vi "运维调试_五参数.vi"() -> ()   [LabVIEW 2016, in "斯坦道多参数.lvlib"]
uses:
  <vilib>/Utility/miscctls.llb/LVPointTypeDef.ctl
  <vilib>/Utility/config.llb/NI_LVConfig.lvlib
panel:
  in  "获取传感器参数并保存触发":bool
  in  "传感器参数自动获取":bool=TRUE
  in  "标样测试组数":dbl=1.0 caption="标样测试组数:"
  in  "水样测试组数":dbl=1.0 caption="水样测试组数:"
  in  "转刷清洗时间":dbl=30.0 caption="转刷清洗时间:"
  in  "上电初始化时间":dbl=5.0 caption="上电初始化时间:"
  in  "水样稳定时间":dbl=5.0 caption="水样稳定时间:"
  out "串口号":string
  in  "水深写入":bool
  in  "水深读取":bool
  in  "水深校准":dbl caption="水深校准:"
  in  "仪器参数设置":bool
  out "模块版本号":string
  in  "写入":bool
  in  "读取":bool
  in  "B":dbl caption="校准值B:"
  in  "K":dbl caption="校准值K:"
  in  "标样核查":bool
  in  "串口设置":bool
  in  "质控参数设置":bool
  in  "打开串口":bool
  in  "释放串口":bool
  out "多参数横条运行状态":T1(xcontrol)
  in  "数据区":i32(listbox)
  in  "停止测量(单探)":bool
  in  "启动测量(单探)":bool
  in  "控制命令区探头选择":u16(ring)=9 items=["氨氮"=3, "水温"=9, "pH值"=10, "溶解氧"=11, "电导率"=12, "浊度"=13, "叶绿素a"=14, "藻密度"=15, "蓝绿藻"=16, "氧化还原电位"=17, "溶解氧%"=18, "盐度"=19]
  in  "同步时间":bool
  in  "初始化(清洗)":bool
  in  "停止测量(全部)":bool
  in  "启动测量(全部)":bool
  in  "关键参数区读取":bool
  in  "关键参数区":i32(listbox)
  in  "传感器参数读取":bool
  in  "传感器区":i32(listbox)
  in  "返回":bool
  in  "设置":bool
  out "运行状态":string
  in  "停止":bool
  in  "水样测试":bool
  out "集成报警信息":string
  # "min"
  # "组"
  # "组"
  # "s"
  # "s"
  # "控制命令区"
  # "探头校准"
  # "水深校准"
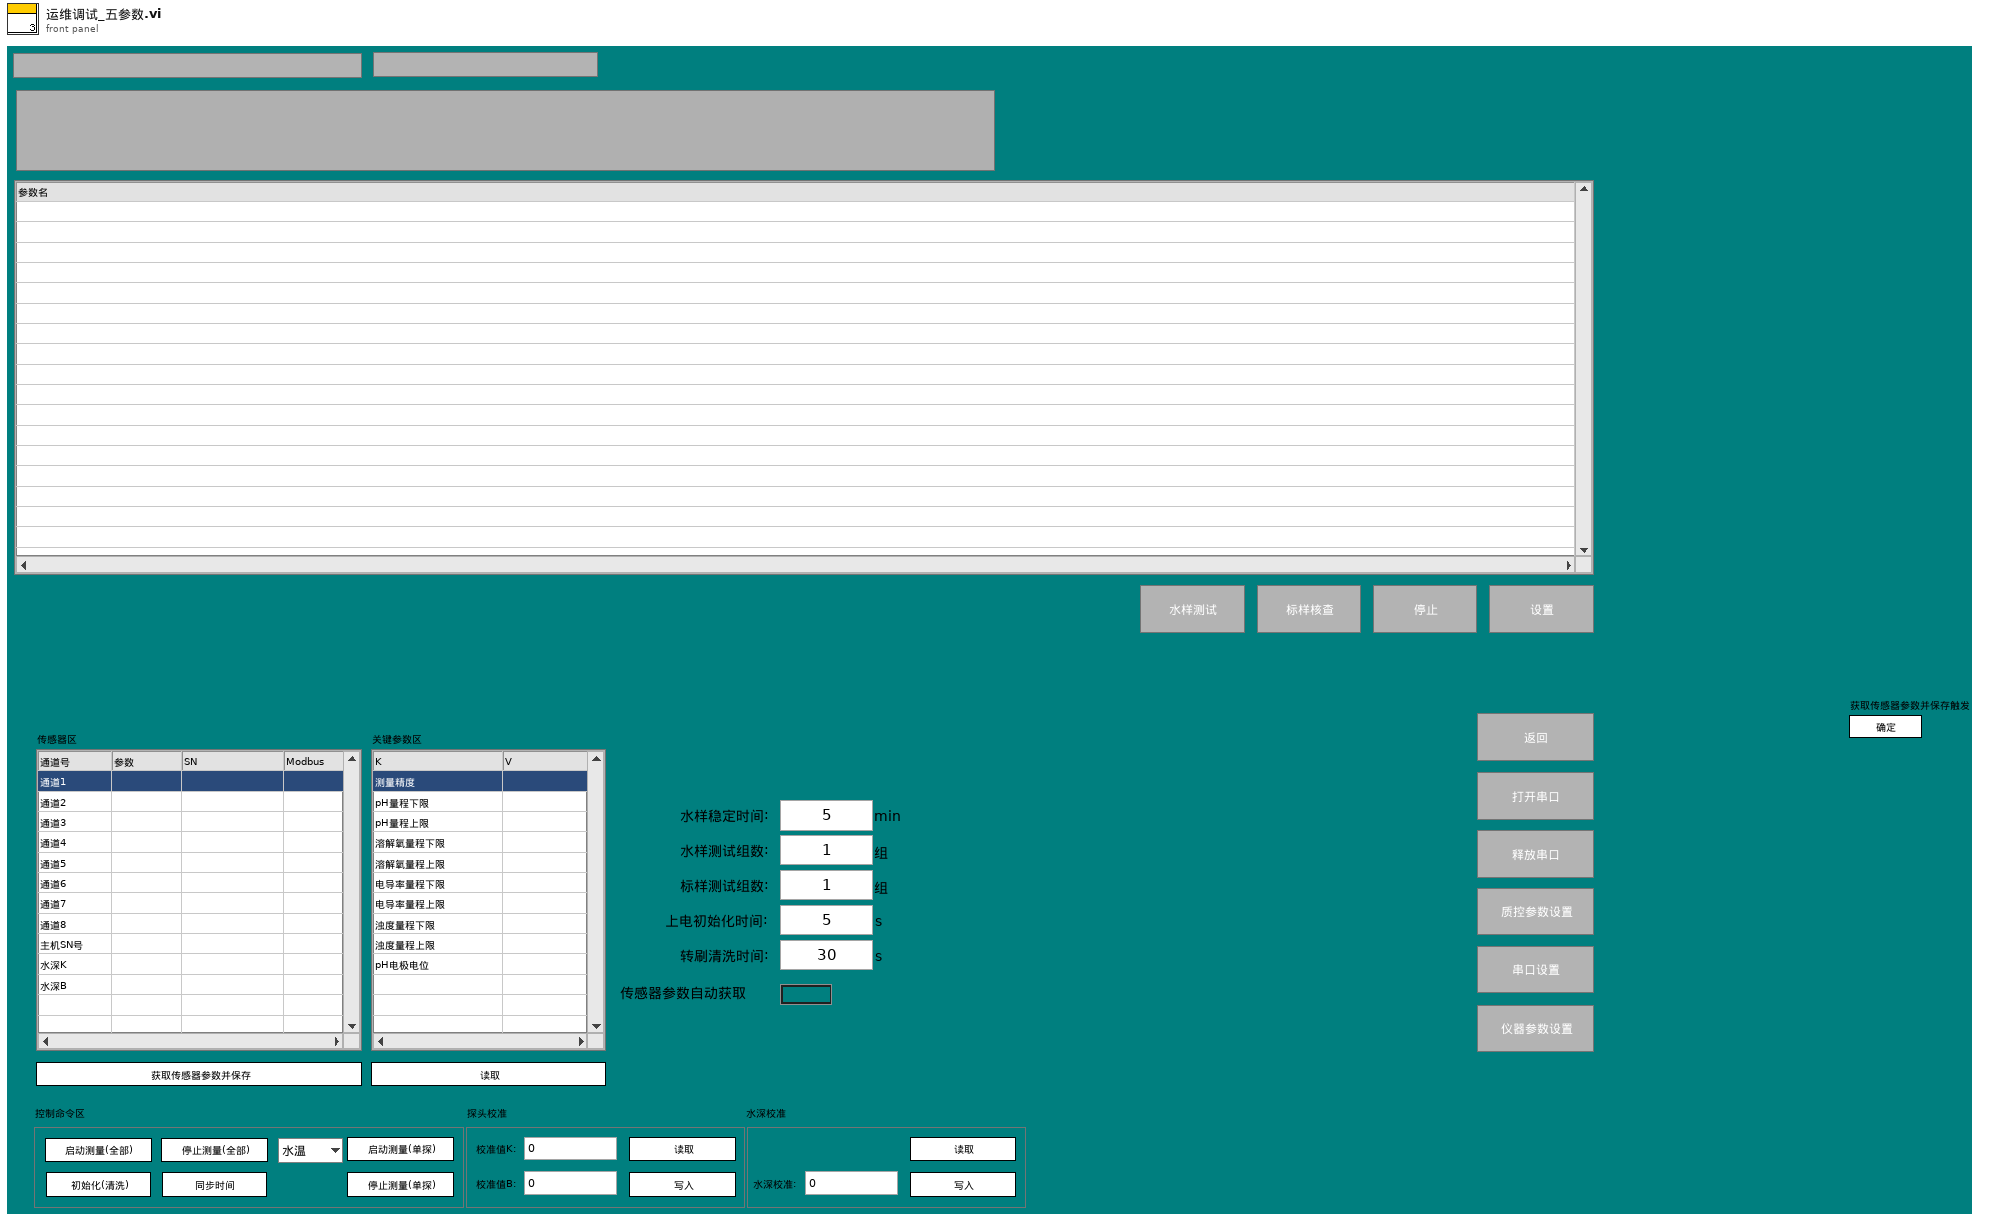
[diagram p1: front panel]
types:
  T1 = cluster{"系统时间":timestamp, "工作状态":u16, "测量模式":u16, "告警代码":enum16{"无告警", "缺试剂告警", "缺水样告警", "缺蒸馏水告警", "缺标液告警", "仪表漏液告警", "标定异常告警", "超量程告警", "加热异常", "低试剂预警", "超上限告警", "超下限告警", "仪表内部其他异常", "滴定异常告警", "电极异常告警", "量程切换告警", "参数设置告警", "PH电极电位异常", "电导率电极异常", "浊度光度异常", "溶解氧电极异常", "溶解氧光强异常", "温度异常告警", "PH异常告警", "溶解氧异常告警", "电导率异常告警", "浊度异常告警", "叶绿素异常告警", "藻密度异常告警", "蓝绿藻异常告警", "ORP异常告警", "氨氮异常告警", "清洁刷异常告警", "SD卡异常告警", "蓝牙异常告警", "Wifi异常告警", "流程异常告警"}, "故障代码":enum16{"无故障", "电机故障", "温度故障", "通讯故障", "滴定故障"}, "日志代码":u16, "软件版本":string}
  T2 = typedef "斯坦道多参数.lvlib/水样测试启动自定义输入参数.ctl" = cluster{"测量模式":enum16{"待机", "水样测试", "标样核查", "零点核查", "跨度核查", "空白测试", "平行样测试", "加标回收", "空白校准", "标样校准", "初始化（清洗）"}, "数据类型":string, "手动启动标记":bool}
  T3 = typedef "LVPointTypeDef.ctl" = cluster{"Horizontal":i16, "Vertical":i16}
  T4 = cluster{"测量量程":dbl, "测量精度":dbl, "测量间隔":dbl, "消解温度":dbl, "消解时长":dbl, "空白校准时间":timestamp, "曲线截距":dbl, "曲线斜率":dbl, "测量检出限":dbl, "测量信号值":dbl, "线性相关系数":dbl, "二次多项式系数":dbl, "标样校准时间":timestamp, "稀释倍数":dbl, "三项式系数":dbl, "空白标定系数":dbl, "量程系数":dbl, "F0/ORPA":dbl, "F1/ORPB":dbl, "F2/ORPK":dbl, "F3":dbl, "F4":dbl, "F5":dbl, "F6":dbl, "F7":dbl, "X0/滴定数":dbl, "量程":dbl}
  T5 = cluster{"因子编码":string, "单位":string, "标样参考值":sgl, "水样数据时间":timestamp, "水样实测值":sgl, "水样数据标识":string, "K":sgl, "B":sgl, "T":sgl, "H":sgl, "水深":sgl, "探头温度":sgl}
  T6 = cluster{"测量量程":dbl, "测量精度":dbl, "测量间隔":dbl, "消解温度":dbl, "消解时长":dbl, "空白校准时间":timestamp, "曲线截距":dbl, "曲线斜率":dbl, "测量检出限":dbl, "测量信号值":dbl, "线性相关系数":dbl, "二次多项式系数":dbl, "标样校准时间":timestamp, "稀释倍数":dbl, "三项式系数":dbl, "空白标定系数":dbl, "量程系数":dbl, "F0/ORPA":dbl, "F1/ORPB":dbl, "F2/ORPK":dbl, "F3":dbl, "F4":dbl, "F5":dbl, "F6":dbl, "F7":dbl, "X0/滴定数":dbl, "量程":dbl}[]
  T7 = cluster{"因子编码":string, "单位":string, "标样参考值":sgl, "水样数据时间":timestamp, "水样实测值":sgl, "水样数据标识":string, "K":sgl, "B":sgl, "T":sgl, "H":sgl, "水深":sgl, "探头温度":sgl}[]
  T8 = cluster{"时间标识":timestamp, "设备":string, "日志信息":string}
  T9 = enum16{"无告警", "缺试剂告警", "缺水样告警", "缺蒸馏水告警", "缺标液告警", "仪表漏液告警", "标定异常告警", "超量程告警", "加热异常", "低试剂预警", "超上限告警", "超下限告警", "仪表内部其他异常", "滴定异常告警", "电极异常告警", "量程切换告警", "参数设置告警", "PH电极电位异常", "电导率电极异常", "浊度光度异常", "溶解氧电极异常", "溶解氧光强异常", "温度异常告警", "PH异常告警", "溶解氧异常告警", "电导率异常告警", "浊度异常告警", "叶绿素异常告警", "藻密度异常告警", "蓝绿藻异常告警", "ORP异常告警", "氨氮异常告警", "清洁刷异常告警", "SD卡异常告警", "蓝牙异常告警", "Wifi异常告警", "流程异常告警"}
  T10 = cluster{"水温":dbl, "pH":dbl, "DO":dbl, "Cond":dbl, "Turb":dbl, "叶绿素":dbl, "藻密度":dbl, "蓝绿藻":dbl, "ORP":dbl, "NH3N":dbl}
  T11 = cluster{"Major":u16, "Minor":u16, "Fix":u16, "Build":u16}
  T12 = typedef "NI_LVConfig.lvlib/Config Data RefNum.ctl" = refnum<k1>
  T13 = enum8{"Enabled", "Disabled", "Disabled and Grayed Out"}
  T14 = typedef "斯坦道多参数.lvlib/标样核查启动自定义输入参数.ctl" = cluster{"测量模式":enum16{"待机", "水样测试", "标样核查", "零点核查", "跨度核查", "空白测试", "平行样测试", "加标回收", "空白校准", "标样校准", "初始化（清洗）"}, "数据标记表":string, "输出参数":cluster{"水温":bool, "pH":bool, "DO":bool, "浊度":bool, "电导率":bool}}
  T15 = cluster{"水温标准液标准浓度":dbl, "酸碱度标准液标准浓度":dbl, "溶解氧标准液标准浓度":dbl, "电导率标准液标准浓度":dbl, "浊度标准液标准浓度":dbl}
  T16 = cluster{"确定":bool, "水温标准液标准浓度":dbl, "酸碱度标准液标准浓度":dbl, "溶解氧标准液标准浓度":dbl, "电导率标准液标准浓度":dbl, "浊度标准液标准浓度":dbl}
  T17 = cluster{"运行模式":enum16{"维护模式", "常规模式", "应急模式", "质控模式"}, "24H周期设置":bool[]}
  T18 = cluster{"水温":bool, "pH":bool, "DO":bool, "浊度":bool, "电导率":bool}
  T19 = enum32{"Bad", "Idle", "Run top level", "Running"}
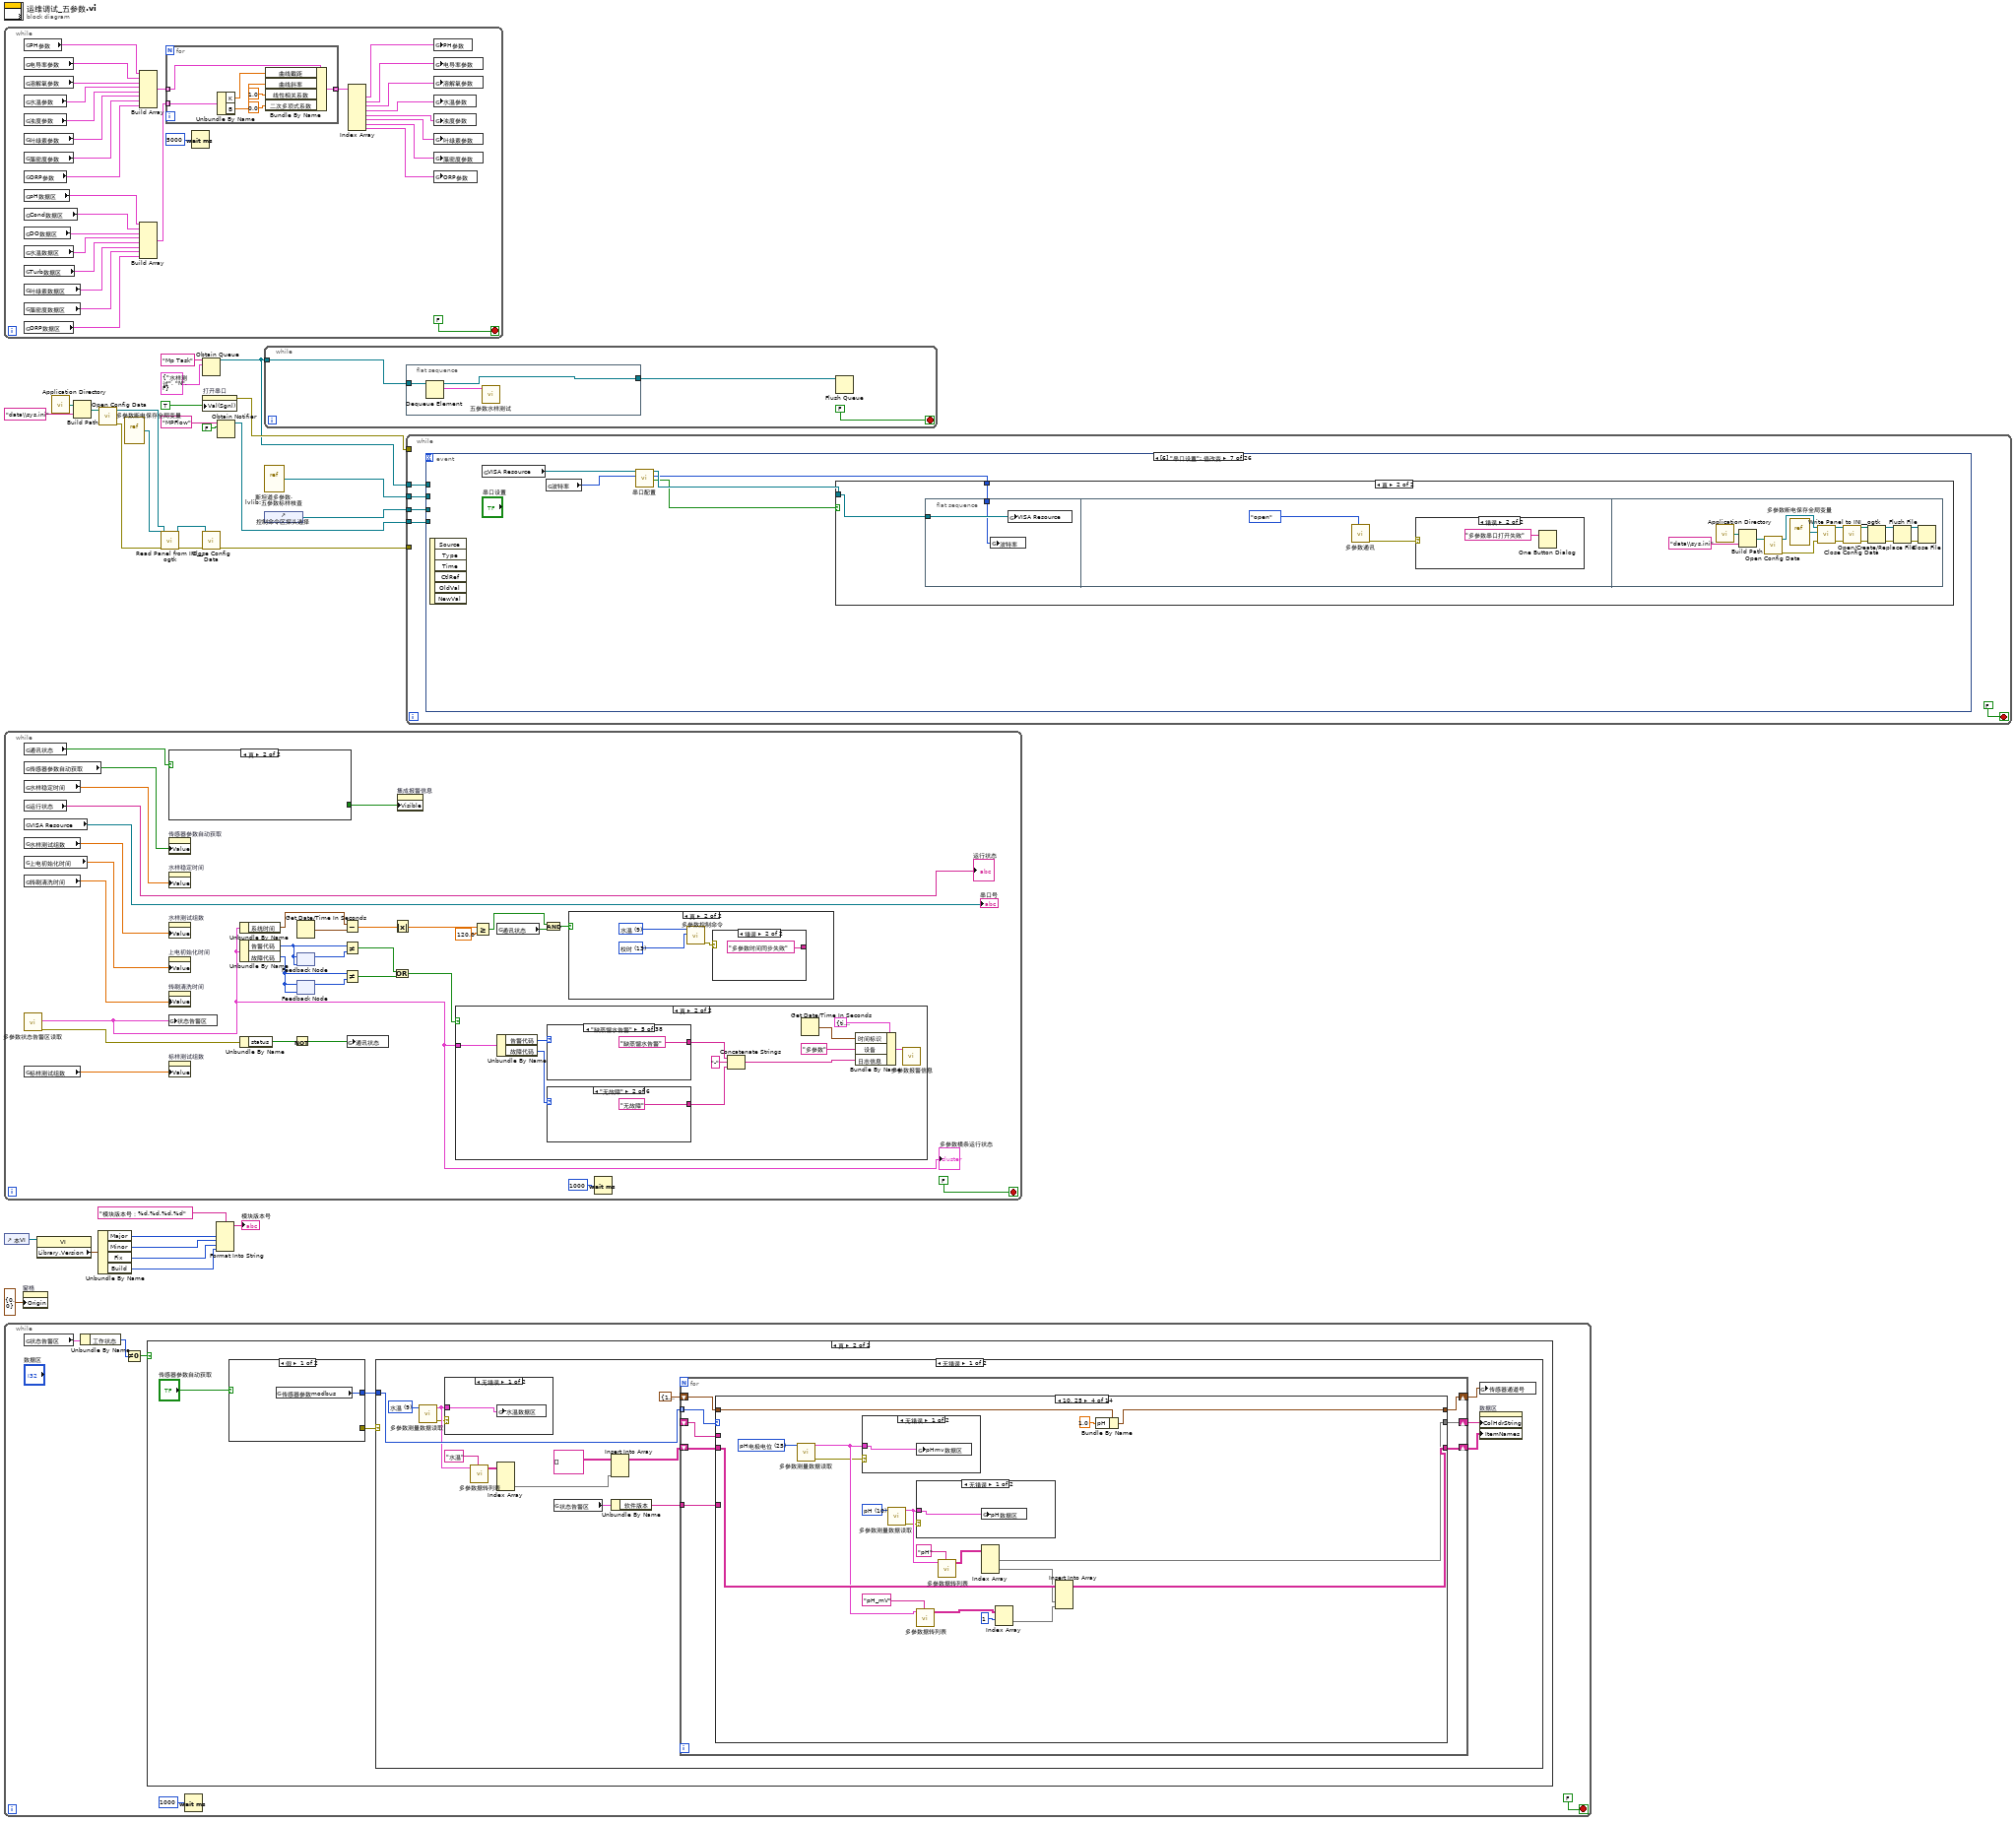
[diagram p0: block diagram]
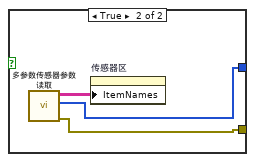
[diagram p3: hidden frame]
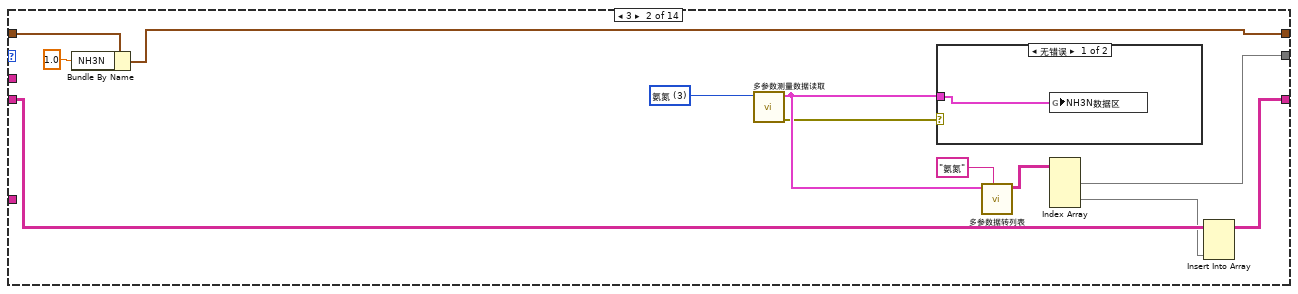
[diagram p6: hidden frame]
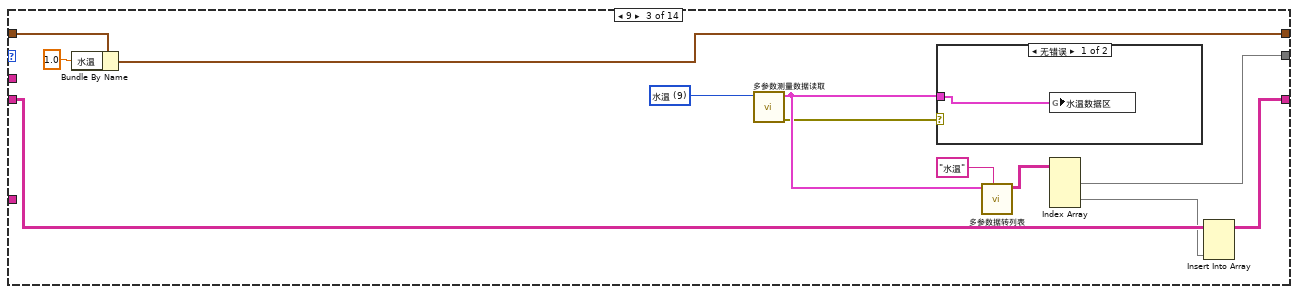
[diagram p8: hidden frame]
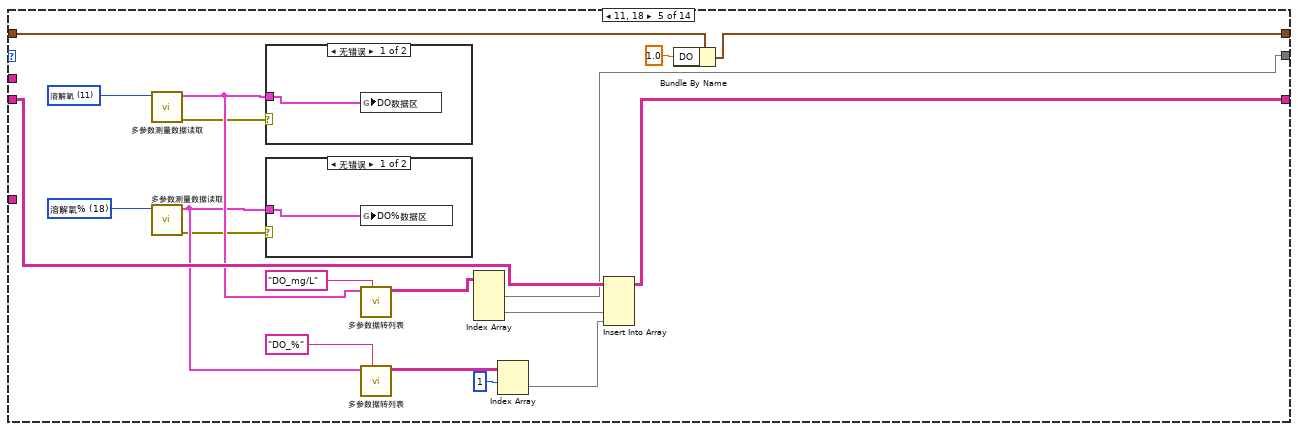
[diagram p12: hidden frame]
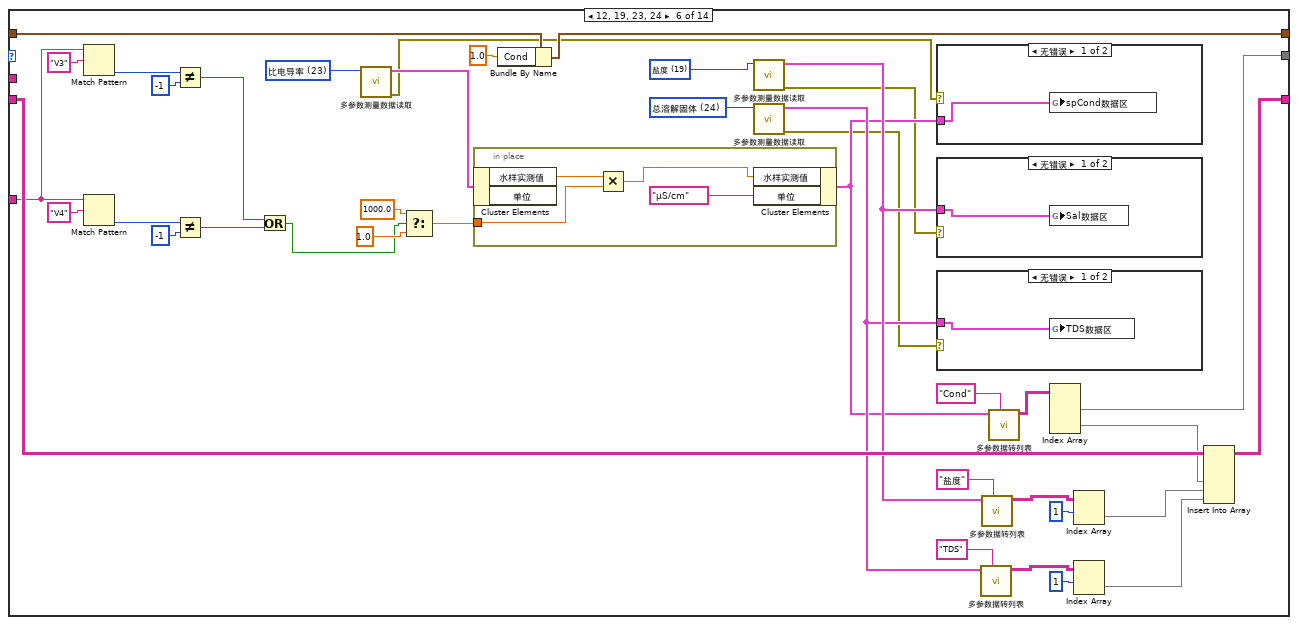
[diagram p15: hidden frame]
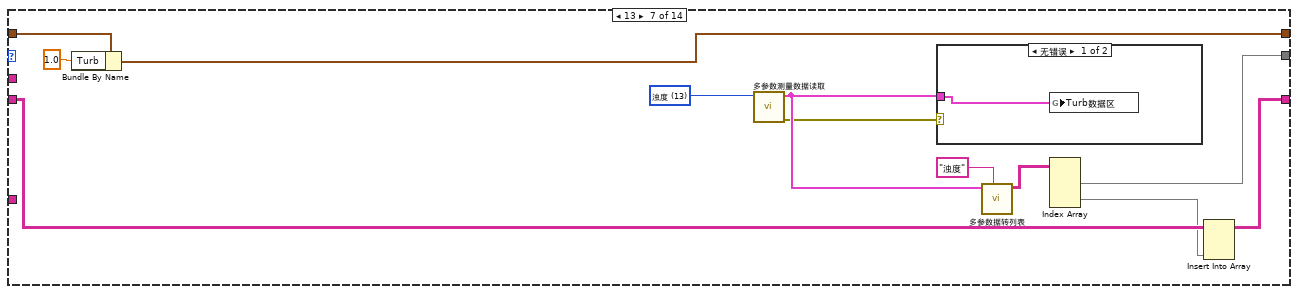
[diagram p19: hidden frame]
diagram:
  n1 = while {
    stop <- FALSE stop-if-true
    n2 = global read "多参数断电保存全局变量.vi" "PH参数"() -> (w47:T4)
    n3 = global read "多参数断电保存全局变量.vi" "电导率参数"() -> (w46:T4)
    n4 = global read "多参数断电保存全局变量.vi" "溶解氧参数"() -> (w45:T4)
    n5 = global read "多参数断电保存全局变量.vi" "水温参数"() -> (w44:T4)
    n6 = global read "多参数断电保存全局变量.vi" "浊度参数"() -> (w43:T4)
    n7 = global read "多参数断电保存全局变量.vi" "叶绿素参数"() -> (w42:T4)
    n8 = global read "多参数断电保存全局变量.vi" "藻密度参数"() -> (w41:T4)
    n9 = global read "多参数断电保存全局变量.vi" "ORP参数"() -> (w40:T4)
    n10 = global read "多参数全局变量.vi" "pH数据区"() -> (w55:T5)
    n11 = global read "多参数全局变量.vi" "Cond数据区"() -> (w54:T5)
    n12 = global read "多参数全局变量.vi" "DO数据区"() -> (w53:T5)
    n13 = global read "多参数全局变量.vi" "水温数据区"() -> (w52:T5)
    n14 = global read "多参数全局变量.vi" "Turb数据区"() -> (w51:T5)
    n15 = global read "多参数全局变量.vi" "叶绿素数据区"() -> (w50:T5)
    n16 = global read "多参数全局变量.vi" "藻密度数据区"() -> (w49:T5)
    n17 = global read "多参数全局变量.vi" "ORP数据区"() -> (w48:T5)
    n18 = Build Array(w47, w46, w45, w44, w43, w42, w41, w40) -> (w39:T6)
    n19 = Build Array(w55, w54, w53, w52, w51, w50, w49, w48) -> (w38:T7)
    n20 = for {
      tunnel: w39 -> [w60] mode=indexing
      tunnel: w38 -> [w59] mode=indexing
      tunnel: [w58] -> w37 mode=indexing
      n21 = Unbundle By Name(w59) -> ("K"=w64:sgl, "B"=w63:sgl)
      n22 = Bundle By Name(cluster=w60, "曲线截距"=w64, "曲线斜率"=w63, "线性相关系数"=1.0, "二次多项式系数"=0.0) -> (w58:T4)
    }
    n23 = Wait (ms)(milliseconds to wait=u32 5000 ("等待时间（毫秒）")) -> ()  [unwired: 1 out]
    n24 = Index Array(array=w37) -> (element #1=w36:T4, element #2=w35:T4, element #3=w34:T4, element #4=w33:T4, element #5=w32:T4, element #6=w31:T4, element #7=w30:T4, element #8=w29:T4)  [unwired: 8 in]
    n25 = global write "多参数断电保存全局变量.vi" "PH参数"(w36) -> ()
    n26 = global write "多参数断电保存全局变量.vi" "电导率参数"(w35) -> ()
    n27 = global write "多参数断电保存全局变量.vi" "溶解氧参数"(w34) -> ()
    n28 = global write "多参数断电保存全局变量.vi" "水温参数"(w33) -> ()
    n29 = global write "多参数断电保存全局变量.vi" "浊度参数"(w32) -> ()
    n30 = global write "多参数断电保存全局变量.vi" "叶绿素参数"(w31) -> ()
    n31 = global write "多参数断电保存全局变量.vi" "藻密度参数"(w30) -> ()
    n32 = global write "多参数断电保存全局变量.vi" "ORP参数"(w29) -> ()
  }
  n33 = while {
    stop <- FALSE stop-if-true
    n34 = global read "多参数全局变量.vi" "通讯状态"() -> (w93:bool)
    n35 = global read "多参数断电保存全局变量.vi" "传感器参数自动获取"() -> (w65:bool)
    n36 = global read "多参数断电保存全局变量.vi" "水样稳定时间"() -> (w70:dbl)
    n37 = global read "多参数全局变量.vi" "运行状态"() -> (→"运行状态":string)
    n38 = global read "多参数断电保存全局变量.vi" "VISA Resource"() -> (→"串口号":refnum<visa-resource-name>)
    n39 = global read "多参数断电保存全局变量.vi" "水样测试组数"() -> (w69:dbl)
    n40 = global read "多参数断电保存全局变量.vi" "上电初始化时间"() -> (w68:dbl)
    n41 = global read "多参数断电保存全局变量.vi" "转刷清洗时间"() -> (w67:dbl)
    n42 = call "多参数状态告警区读取.vi"() -> ("error out"=w83:errorcluster, "状态告警块"=w80:T1)  [unwired: 9 in, 1 out]
    "多参数横条运行状态" <- w80
    n43 = global read "多参数断电保存全局变量.vi" "标样测试组数"() -> (w66:dbl)
    n44 = case shown="真" w93 {
      tunnel: [TRUE ("可见") _] -> w92
      frame False {
        "集成报警信息" <- "通讯异常" ("集成报警信息")
      }
      frame True {
      }
    }
    n45 = property on="传感器参数自动获取" class="Bool (严格)"("Value"=w65) -> ()  [unwired: 2 in, 2 out]
    n46 = property on="水样稳定时间" class="DigNum (严格)"("Value"=w70) -> ()  [unwired: 2 in, 2 out]
    n47 = property on="水样测试组数" class="DigNum (严格)"("Value"=w69) -> ()  [unwired: 2 in, 2 out]
    n48 = property on="上电初始化时间" class="DigNum (严格)"("Value"=w68) -> ()  [unwired: 2 in, 2 out]
    n49 = property on="转刷清洗时间" class="DigNum (严格)"("Value"=w67) -> ()  [unwired: 2 in, 2 out]
    n50 = global write "多参数全局变量.vi" "状态告警区"(w80) -> ()
    n51 = property on="标样测试组数" class="DigNum (严格)"("Value"=w66) -> ()  [unwired: 2 in, 2 out]
    n52 = Unbundle By Name(w80) -> ("系统时间"=w79:timestamp)
    n53 = Unbundle By Name(w80) -> ("告警代码"=w89:T9, "故障代码"=w87:enum16{"无故障", "电机故障", "温度故障", "通讯故障", "滴定故障"})
    n54 = Unbundle By Name(w83) -> ("status"=w82:bool)
    n55 = Not(x=w82) -> (.not. x?=w81:bool)
    n56 = Get Date/Time In Seconds() -> (seconds since 1Jan1904=w78:timestamp)
    n57 = feedback #1(w89) -> (w90:T9)
    n58 = feedback-in #1(w89) -> ()
    n59 = feedback #2(w87) -> (w88:enum16{"无故障", "电机故障", "温度故障", "通讯故障", "滴定故障"})
    n60 = feedback-in #2(w87) -> ()
    n61 = Subtract(x=w79, y=w78) -> (x-y=w77:dbl)
    n62 = Not Equal?(x=w89, y=w90) -> (x != y?=w85:bool)
    n63 = Not Equal?(x=w87, y=w88) -> (x != y?=w86:bool)
    n64 = global write "多参数全局变量.vi" "通讯状态"(w81) -> ()
    n65 = Absolute Value(x=w77) -> (abs(x)=w76:dbl)
    n66 = Or(x=w85, y=w86) -> (x .or. y?=w84:bool)
    n67 = property on="集成报警信息" class="Str"("Visible"=w92) -> ()  [unwired: 2 in, 2 out]
    n68 = case shown="真" w84 {
      tunnel: w80 -> [_ w111]
      frame False {
      }
      frame True {
        n69 = Unbundle By Name(w111) -> ("告警代码"=w110:T9, "故障代码"=w109:enum16{"无故障", "电机故障", "温度故障", "通讯故障", "滴定故障"})
        n70 = case shown="\"缺蒸馏水告警\"" w110 {
          selector: w110 -> [w122 _ _ _ _ _ _ _ _ _ _ _ _ _ _ _ _ _ _ _ _ _ _ _ _ _ _ _ _ _ _ _ _ _ _ _ _ _]
          tunnel: [w121 "无告警" "缺试剂告警" "缺水样告警" "缺蒸馏水告警" "缺标液告警" "仪表漏液告警" "标定异常告警" "超量程告警" "加热异常" "低试剂预警" "超上限告警" "超下限告警" "仪表内部其他异常" "滴定异常告警" "电极异常告警" "量程切换告警" "参数设置告警" "PH电极电位异常" "电导率电极异常" "浊度光度异常" "溶解氧电极异常" "溶解氧光强异常" "温度异常告警" "PH异常告警" "溶解氧异常告警" "电导率异常告警" "浊度异常告警" "叶绿素异常告警" "藻密度异常告警" "蓝绿藻异常告警" "ORP异常告警" "氨氮异常告警" "清洁刷异常告警" "SD卡异常告警" "蓝牙异常告警" "WiFi异常告警" "流程异常告警"] -> w108
          frame Default {
            n71 = Format Into String(format string="%d" ("格式字符串"), initial string="未知" ("工作状态"), w122) -> (resulting string=w121:string)  [unwired: 1 in, 1 out]
          }
          frame "无告警" {
          }
          frame "缺试剂告警" {
          }
          frame "缺水样告警" {
          }
          frame "缺蒸馏水告警" {
          }
          frame "缺标液告警" {
          }
          frame "仪表漏液告警" {
          }
          frame "标定异常告警" {
          }
          frame "超量程告警" {
          }
          frame "加热异常" {
          }
          frame "低试剂预警" {
          }
          frame "超上限告警" {
          }
          frame "超下限告警" {
          }
          frame "仪表内部其他异常" {
          }
          frame "滴定异常告警" {
          }
          frame "电极异常告警" {
          }
          frame "量程切换告警" {
          }
          frame "参数设置告警" {
          }
          frame "PH电极电位异常" {
          }
          frame "电导率电极异常" {
          }
          frame "浊度光度异常" {
          }
          frame "溶解氧电极异常" {
          }
          frame "溶解氧光强异常" {
          }
          frame "温度异常告警" {
          }
          frame "PH异常告警" {
          }
          frame "溶解氧异常告警" {
          }
          frame "电导率异常告警" {
          }
          frame "浊度异常告警" {
          }
          frame "叶绿素异常告警" {
          }
          frame "藻密度异常告警" {
          }
          frame "蓝绿藻异常告警" {
          }
          frame "ORP异常告警" {
          }
          frame "氨氮异常告警" {
          }
          frame "清洁刷异常告警" {
          }
          frame "SD卡异常告警" {
          }
          frame "蓝牙异常告警" {
          }
          frame "Wifi异常告警" {
          }
          frame "流程异常告警" {
          }
        }
        n72 = case shown="\"无故障\"" w109 {
          selector: w109 -> [w113 _ _ _ _ _]
          tunnel: [w112 "无故障" "电机故障" "温度故障" "通讯故障" "滴定故障"] -> w107
          frame Default {
            n73 = Format Into String(format string="%d" ("格式字符串"), initial string="未知" ("工作状态"), w113) -> (resulting string=w112:string)  [unwired: 1 in, 1 out]
          }
          frame "无故障" {
          }
          frame "电机故障" {
          }
          frame "温度故障" {
          }
          frame "通讯故障" {
          }
          frame "滴定故障" {
          }
        }
        n74 = Concatenate Strings(w108, "-" ("字符串"), w107) -> (w103:string)
        n75 = Get Date/Time In Seconds() -> (seconds since 1Jan1904=w102:timestamp)
        n76 = Bundle By Name(cluster=T8 {"时间标识"=timestamp(0 s since 1904-01-01), "设备"="", "日志信息"=""} ("data in"), "时间标识"=w102, "设备"="多参数", "日志信息"=w103) -> (w104:T8)
        n77 = call "多参数报警信息.vi"("data in"=w104) -> ()  [unwired: 10 in, 1 out]
      }
    }
    n78 = Greater Or Equal?(x=w76, y=120.0) -> (x >= y?=w75:bool)
    n79 = global read "多参数全局变量.vi" "通讯状态"() -> (w72:bool)
    n80 = And(x=w75, y=w72) -> (x .and. y?=w73:bool)
    n81 = case shown="真" w73 {
      frame False {
      }
      frame True {
        w96 = u16 13 items=["启动测量（全部）"=1, "初始化（清洗）"=10, "停止测量（全部）"=11, "校时"=13, "启动测量（单个传感器）"=19, "停止测量（单个传感器）"=20] ("控制命令")
        w97 = u16 9 items=["氨氮"=3, "水温"=9, "pH值"=10, "溶解氧"=11, "电导率"=12, "浊度"=13, "叶绿素a"=14, "藻密度"=15, "蓝绿藻"=16, "氧化还原电位"=17, "溶解氧%"=18, "盐度"=19] ("站号")
        n82 = call "多参数控制命令.vi"("控制命令"=w96, "站号"=w97) -> ("error out"=w98:errorcluster)  [unwired: 9 in]
        n83 = case shown="错误" w98 {
          tunnel: ["多参数时间同步成功" ("消息") "多参数时间同步失败" ("消息")] -> _
          frame No Error {
          }
          frame Error {
          }
        }
      }
    }
    n84 = Wait (ms)(milliseconds to wait=u32 1000 ("等待时间（毫秒）")) -> ()  [unwired: 1 out]
  }
  n85 = control-ref of="本VI"() -> (w8:refnum<vi>)
  n86 = while {
    stop <- FALSE stop-if-true
    n87 = global read "多参数全局变量.vi" "状态告警区"() -> (w166:T1)
    n88 = Unbundle By Name(w166) -> ("工作状态"=w165:u16)
    n89 = Not Equal To 0?(x=w165) -> (x != 0?=w164:bool)
    n90 = case shown="真" w164 {
      frame False {
      }
      frame True {
        n91 = case shown="假" "传感器参数自动获取" {
          tunnel: [_ w175] -> w171
          tunnel: [w172 w174] -> w170
          frame False {
            n92 = global read "多参数断电保存全局变量.vi" "传感器参数modbus"() -> (w172:u16[])
          }
          frame True {
            n93 = call "多参数传感器参数读取.vi"() -> ("error out"=w175:errorcluster, "modbus"=w174:u16[], "添加的数组"=w173:string[][])  [unwired: 9 in]
            n94 = property on="传感器区" class="MCListbox (严格)"("ItemNames"=w173) -> ()  [unwired: 2 in, 2 out]
          }
        }
        n95 = case shown="无错误" w171 {
          tunnel: w170 -> [w190 _]
          frame No Error {
            w187 = u16 9 items=["氨氮"=3, "水温"=9, "pH"=10, "溶解氧"=11, "电导率"=12, "浊度"=13, "叶绿素a"=14, "藻密度"=15, "蓝绿藻"=16, "氧化还原电位"=17, "溶解氧%"=18, "盐度"=19, "水中油"=20, "高锰酸盐指数"=21, "化学需氧量"=22, "比电导率"=23, "总溶解固体"=24, "pH电极电位"=25] ("下拉列表")
            n96 = call "多参数测量数据读取.vi"("探头选择"=w187) -> ("error out"=w176:errorcluster, "测量数据块"=w182:T5)  [unwired: 8 in, 1 out]
            n97 = case shown="无错误" w176 {
              tunnel: w182 -> [w191 _]
              frame No Error {
                n98 = global write "多参数全局变量.vi" "水温数据区"(w191) -> ()
              }
              frame Error {
              }
            }
            n99 = call "多参数据转列表.vi"("参数名"="水温", "测量数据块"=w182) -> ("添加的数组"=w180:string[][])  [unwired: 9 in]
            n100 = Index Array(array=w180) -> (element #2=w179:string[])  [unwired: 4 in, 1 out]
            n101 = global read "多参数全局变量.vi" "状态告警区"() -> (w178:T1)
            n102 = Insert Into Array(array=string[][] [] ("子数组"), new element=w179) -> (w185:string[][])  [unwired: 2 in]
            n103 = Unbundle By Name(w178) -> ("软件版本"=w177:string)
            n104 = for {
              tunnel: w190 -> [w199] mode=indexing
              shift-right: [w197] -> w188
              shift-left: w185 -> [w198]
              shift-right: [w196] -> w189
              shift-left: _ -> [w195]
              shift-right: [w194] -> w183
              shift-left: T10 {"水温"=1.0, "pH"=0.0, "DO"=0.0, "Cond"=0.0, "Turb"=0.0, "叶绿素"=0.0, "藻密度"=0.0, "蓝绿藻"=0.0, "ORP"=0.0, "NH3N"=0.0} ("传感器通道号") -> [w193]
              tunnel: w177 -> [w192]
              n105 = case shown="10, 25" w199 {
                tunnel: w198 -> [w202 w213 w226 w246 w267 w309 w328 w341 w354 w367 w380 w390 w399 w408]
                tunnel: [w202 w212 w225 w245 w266 w308 w327 w340 w353 w366 w379 w389 w398 w407] -> w197
                tunnel: [w201 w205 w218 w238 w259 w300 w321 w333 w348 w360 w373 w384 w393 w402] -> w196
                tunnel: w195 -> [w201 _ _ _ _ _ _ _ _ _ _ _ _ _]
                tunnel: [w200 w209 w222 w241 w263 w303 w324 w337 w350 w363 w376 w388 w397 w406] -> w194
                tunnel: w193 -> [w200 w211 w224 w243 w265 w304 w325 w338 w351 w364 w377 w388 w397 w406]
                tunnel: w192 -> [_ _ _ _ _ w279 _ _ _ _ _ _ _ _]
                frame 0, Default {
                }
                frame 3 {
                  w214 = u16 3 items=["氨氮"=3, "水温"=9, "pH"=10, "溶解氧"=11, "电导率"=12, "浊度"=13, "叶绿素a"=14, "藻密度"=15, "蓝绿藻"=16, "氧化还原电位"=17, "溶解氧%"=18, "盐度"=19, "水中油"=20, "高锰酸盐指数"=21, "化学需氧量"=22, "比电导率"=23, "总溶解固体"=24, "pH电极电位"=25] ("下拉列表")
                  n106 = Bundle By Name(cluster=w211, "NH3N"=1.0) -> (w209:T10)
                  n107 = call "多参数测量数据读取.vi"("探头选择"=w214) -> ("error out"=w203:errorcluster, "测量数据块"=w208:T5)  [unwired: 8 in, 1 out]
                  n108 = case shown="无错误" w203 {
                    tunnel: w208 -> [w215 _]
                    frame No Error {
                      n109 = global write "多参数全局变量.vi" "NH3N数据区"(w215) -> ()
                    }
                    frame Error {
                    }
                  }
                  n110 = call "多参数据转列表.vi"("参数名"="氨氮", "测量数据块"=w208) -> ("添加的数组"=w207:string[][])  [unwired: 9 in]
                  n111 = Index Array(array=w207) -> (element #1=w205:string[], element #2=w204:string[])  [unwired: 4 in]
                  n112 = Insert Into Array(array=w213, new element=w204) -> (w212:string[][])  [unwired: 2 in]
                }
                frame 9 {
                  w227 = u16 9 items=["氨氮"=3, "水温"=9, "pH"=10, "溶解氧"=11, "电导率"=12, "浊度"=13, "叶绿素a"=14, "藻密度"=15, "蓝绿藻"=16, "氧化还原电位"=17, "溶解氧%"=18, "盐度"=19, "水中油"=20, "高锰酸盐指数"=21, "化学需氧量"=22, "比电导率"=23, "总溶解固体"=24, "pH电极电位"=25] ("下拉列表")
                  n113 = Bundle By Name(cluster=w224, "水温"=1.0) -> (w222:T10)
                  n114 = call "多参数测量数据读取.vi"("探头选择"=w227) -> ("error out"=w216:errorcluster, "测量数据块"=w221:T5)  [unwired: 8 in, 1 out]
                  n115 = case shown="无错误" w216 {
                    tunnel: w221 -> [w228 _]
                    frame No Error {
                      n116 = global write "多参数全局变量.vi" "水温数据区"(w228) -> ()
                    }
                    frame Error {
                    }
                  }
                  n117 = call "多参数据转列表.vi"("参数名"="水温", "测量数据块"=w221) -> ("添加的数组"=w220:string[][])  [unwired: 9 in]
                  n118 = Index Array(array=w220) -> (element #1=w218:string[], element #2=w217:string[])  [unwired: 4 in]
                  n119 = Insert Into Array(array=w226, new element=w217) -> (w225:string[][])  [unwired: 2 in]
                }
                frame 10, 25 {
                  w244 = u16 25 items=["氨氮"=3, "水温"=9, "pH"=10, "溶解氧"=11, "电导率"=12, "浊度"=13, "叶绿素a"=14, "藻密度"=15, "蓝绿藻"=16, "氧化还原电位"=17, "溶解氧%"=18, "盐度"=19, "水中油"=20, "高锰酸盐指数"=21, "化学需氧量"=22, "比电导率"=23, "总溶解固体"=24, "pH电极电位"=25] ("下拉列表")
                  w247 = u16 10 items=["氨氮"=3, "水温"=9, "pH"=10, "溶解氧"=11, "电导率"=12, "浊度"=13, "叶绿素a"=14, "藻密度"=15, "蓝绿藻"=16, "氧化还原电位"=17, "溶解氧%"=18, "盐度"=19, "水中油"=20, "高锰酸盐指数"=21, "化学需氧量"=22, "比电导率"=23, "总溶解固体"=24, "pH电极电位"=25] ("下拉列表")
                  n120 = call "多参数测量数据读取.vi"("探头选择"=w244) -> ("error out"=w229:errorcluster, "测量数据块"=w234:T5)  [unwired: 8 in, 1 out]
                  n121 = case shown="无错误" w229 {
                    tunnel: w234 -> [w248 _]
                    frame No Error {
                      n122 = global write "多参数全局变量.vi" "pHmv数据区"(w248) -> ()
                    }
                    frame Error {
                    }
                  }
                  n123 = call "多参数测量数据读取.vi"("探头选择"=w247) -> ("error out"=w230:errorcluster, "测量数据块"=w240:T5)  [unwired: 8 in, 1 out]
                  n124 = case shown="无错误" w230 {
                    tunnel: w240 -> [w249 _]
                    frame No Error {
                      n125 = global write "多参数全局变量.vi" "pH数据区"(w249) -> ()
                    }
                    frame Error {
                    }
                  }
                  n126 = call "多参数据转列表.vi"("参数名"="pH_mV", "测量数据块"=w234) -> ("添加的数组"=w233:string[][])  [unwired: 9 in]
                  n127 = call "多参数据转列表.vi"("参数名"="pH", "测量数据块"=w240) -> ("添加的数组"=w239:string[][])  [unwired: 9 in]
                  n128 = Index Array(array=w239) -> (element #1=w238:string[], element #2=w237:string[])  [unwired: 4 in]
                  n129 = Index Array(array=w233, index (row)=1 ("禁用的索引 (列)")) -> (element=w236:string[])  [unwired: 1 in]
                  n130 = Insert Into Array(array=w246, new element #1=w237, new element #2=w236) -> (w245:string[][])  [unwired: 2 in]
                  n131 = Bundle By Name(cluster=w243, "pH"=1.0) -> (w241:T10)
                }
                frame 11, 18 {
                  w257 = u16 18 items=["氨氮"=3, "水温"=9, "pH"=10, "溶解氧"=11, "电导率"=12, "浊度"=13, "叶绿素a"=14, "藻密度"=15, "蓝绿藻"=16, "氧化还原电位"=17, "溶解氧%"=18, "盐度"=19, "水中油"=20, "高锰酸盐指数"=21, "化学需氧量"=22, "比电导率"=23, "总溶解固体"=24, "pH电极电位"=25] ("下拉列表")
                  w268 = u16 11 items=["氨氮"=3, "水温"=9, "pH"=10, "溶解氧"=11, "电导率"=12, "浊度"=13, "叶绿素a"=14, "藻密度"=15, "蓝绿藻"=16, "氧化还原电位"=17, "溶解氧%"=18, "盐度"=19, "水中油"=20, "高锰酸盐指数"=21, "化学需氧量"=22, "比电导率"=23, "总溶解固体"=24, "pH电极电位"=25] ("下拉列表")
                  n132 = call "多参数测量数据读取.vi"("探头选择"=w268) -> ("error out"=w251:errorcluster, "测量数据块"=w262:T5)  [unwired: 8 in, 1 out]
                  n133 = call "多参数测量数据读取.vi"("探头选择"=w257) -> ("error out"=w250:errorcluster, "测量数据块"=w256:T5)  [unwired: 8 in, 1 out]
                  n134 = case shown="无错误" w251 {
                    tunnel: w262 -> [w270 _]
                    frame No Error {
                      n135 = global write "多参数全局变量.vi" "DO数据区"(w270) -> ()
                    }
                    frame Error {
                    }
                  }
                  n136 = case shown="无错误" w250 {
                    tunnel: w256 -> [w269 _]
                    frame No Error {
                      n137 = global write "多参数全局变量.vi" "DO%数据区"(w269) -> ()
                    }
                    frame Error {
                    }
                  }
                  n138 = call "多参数据转列表.vi"("参数名"="DO_mg/L", "测量数据块"=w262) -> ("添加的数组"=w260:string[][])  [unwired: 9 in]
                  n139 = call "多参数据转列表.vi"("参数名"="DO_%", "测量数据块"=w256) -> ("添加的数组"=w254:string[][])  [unwired: 9 in]
                  n140 = Index Array(array=w260) -> (element #1=w259:string[], element #2=w258:string[])  [unwired: 4 in]
                  n141 = Index Array(array=w254, index (row)=1 ("禁用的索引 (列)")) -> (element=w253:string[])  [unwired: 1 in]
                  n142 = Insert Into Array(array=w267, new element #1=w258, new element #2=w253) -> (w266:string[][])  [unwired: 2 in]
                  n143 = Bundle By Name(cluster=w265, "DO"=1.0) -> (w263:T10)
                }
                frame 12, 19, 23, 24 {
                  w306 = u16 24 items=["氨氮"=3, "水温"=9, "pH"=10, "溶解氧"=11, "电导率"=12, "浊度"=13, "叶绿素a"=14, "藻密度"=15, "蓝绿藻"=16, "氧化还原电位"=17, "溶解氧%"=18, "盐度"=19, "水中油"=20, "高锰酸盐指数"=21, "化学需氧量"=22, "比电导率"=23, "总溶解固体"=24, "pH电极电位"=25] ("下拉列表")
                  w307 = u16 19 items=["氨氮"=3, "水温"=9, "pH"=10, "溶解氧"=11, "电导率"=12, "浊度"=13, "叶绿素a"=14, "藻密度"=15, "蓝绿藻"=16, "氧化还原电位"=17, "溶解氧%"=18, "盐度"=19, "水中油"=20, "高锰酸盐指数"=21, "化学需氧量"=22, "比电导率"=23, "总溶解固体"=24, "pH电极电位"=25] ("下拉列表")
                  w310 = u16 23 items=["氨氮"=3, "水温"=9, "pH"=10, "溶解氧"=11, "电导率"=12, "浊度"=13, "叶绿素a"=14, "藻密度"=15, "蓝绿藻"=16, "氧化还原电位"=17, "溶解氧%"=18, "盐度"=19, "水中油"=20, "高锰酸盐指数"=21, "化学需氧量"=22, "比电导率"=23, "总溶解固体"=24, "pH电极电位"=25] ("下拉列表")
                  n144 = Match Pattern(string=w279, regular expression="V3" ("正则表达式")) -> (offset past match=w287:i32)  [unwired: 1 in, 3 out]
                  n145 = Match Pattern(string=w279, regular expression="V4" ("正则表达式")) -> (offset past match=w281:i32)  [unwired: 1 in, 3 out]
                  n146 = Not Equal?(x=w287, y=-1) -> (x != y?=w277:bool)
                  n147 = Not Equal?(x=w281, y=-1) -> (x != y?=w278:bool)
                  n148 = Or(x=w277, y=w278) -> (x .or. y?=w276:bool)
                  n149 = call "多参数测量数据读取.vi"("探头选择"=w310) -> ("error out"=w273:errorcluster, "测量数据块"=w292:T5)  [unwired: 8 in, 1 out]
                  n150 = Select(t=1000.0, s=w276, f=1.0) -> (s? t:f=w283:dbl)
                  n151 = in-place {
                    in-place-border: w283 -> [w314]
                    n152 = in-place-cluster #3(w292) -> ("水样实测值"=w316:sgl)  [unwired: 1 out]
                    n153 = Multiply(x=w316, y=w314) -> (x*y=w315:dbl)
                    n154 = in-place-cluster #3("水样实测值"=w315, "单位"="μS/cm") -> (w291:T5)
                  }
                  n155 = Bundle By Name(cluster=w304, "Cond"=1.0 ("DO")) -> (w303:T10)
                  n156 = call "多参数测量数据读取.vi"("探头选择"=w307) -> ("error out"=w272:errorcluster, "测量数据块"=w297:T5)  [unwired: 8 in, 1 out]
                  n157 = call "多参数测量数据读取.vi"("探头选择"=w306) -> ("error out"=w271:errorcluster, "测量数据块"=w294:T5)  [unwired: 8 in, 1 out]
                  n158 = case shown="无错误" w273 {
                    tunnel: w291 -> [w313 _]
                    frame No Error {
                      n159 = global write "多参数全局变量.vi" "spCond数据区"(w313) -> ()
                    }
                    frame Error {
                    }
                  }
                  n160 = case shown="无错误" w272 {
                    tunnel: w297 -> [w312 _]
                    frame No Error {
                      n161 = global write "多参数全局变量.vi" "Sal数据区"(w312) -> ()
                    }
                    frame Error {
                    }
                  }
                  n162 = case shown="无错误" w271 {
                    tunnel: w294 -> [w311 _]
                    frame No Error {
                      n163 = global write "多参数全局变量.vi" "TDS数据区"(w311) -> ()
                    }
                    frame Error {
                    }
                  }
                  n164 = call "多参数据转列表.vi"("参数名"="TDS", "测量数据块"=w294) -> ("添加的数组"=w293:string[][])  [unwired: 9 in]
                  n165 = call "多参数据转列表.vi"("参数名"="盐度", "测量数据块"=w297) -> ("添加的数组"=w296:string[][])  [unwired: 9 in]
                  n166 = call "多参数据转列表.vi"("参数名"="Cond", "测量数据块"=w291) -> ("添加的数组"=w301:string[][])  [unwired: 9 in]
                  n167 = Index Array(array=w301) -> (element #1=w300:string[], element #2=w299:string[])  [unwired: 4 in]
                  n168 = Index Array(array=w296, index (row)=1 ("禁用的索引 (列)")) -> (element=w275:string[])  [unwired: 1 in]
                  n169 = Index Array(array=w293, index (row)=1 ("禁用的索引 (列)")) -> (element=w274:string[])  [unwired: 1 in]
                  n170 = Insert Into Array(array=w309, new element #1=w299, new element #2=w275, new element #3=w274) -> (w308:string[][])  [unwired: 2 in]
                }
                frame 13 {
                  w329 = u16 13 items=["氨氮"=3, "水温"=9, "pH"=10, "溶解氧"=11, "电导率"=12, "浊度"=13, "叶绿素a"=14, "藻密度"=15, "蓝绿藻"=16, "氧化还原电位"=17, "溶解氧%"=18, "盐度"=19, "水中油"=20, "高锰酸盐指数"=21, "化学需氧量"=22, "比电导率"=23, "总溶解固体"=24, "pH电极电位"=25] ("下拉列表")
                  n171 = Bundle By Name(cluster=w325, "Turb"=1.0 ("DO")) -> (w324:T10)
                  n172 = call "多参数测量数据读取.vi"("探头选择"=w329) -> ("error out"=w318:errorcluster, "测量数据块"=w319:T5)  [unwired: 8 in, 1 out]
                  n173 = case shown="无错误" w318 {
                    tunnel: w319 -> [w330 _]
                    frame No Error {
                      n174 = global write "多参数全局变量.vi" "Turb数据区"(w330) -> ()
                    }
                    frame Error {
                    }
                  }
                  n175 = call "多参数据转列表.vi"("参数名"="浊度", "测量数据块"=w319) -> ("添加的数组"=w322:string[][])  [unwired: 9 in]
                  n176 = Index Array(array=w322) -> (element #1=w321:string[], element #2=w320:string[])  [unwired: 4 in]
                  n177 = Insert Into Array(array=w328, new element=w320) -> (w327:string[][])  [unwired: 2 in]
                }
                frame 14 {
                  w342 = u16 14 items=["氨氮"=3, "水温"=9, "pH"=10, "溶解氧"=11, "电导率"=12, "浊度"=13, "叶绿素a"=14, "藻密度"=15, "蓝绿藻"=16, "氧化还原电位"=17, "溶解氧%"=18, "盐度"=19, "水中油"=20, "高锰酸盐指数"=21, "化学需氧量"=22, "比电导率"=23, "总溶解固体"=24, "pH电极电位"=25] ("下拉列表")
                  n178 = Bundle By Name(cluster=w338, "叶绿素"=1.0 ("DO")) -> (w337:T10)
                  n179 = call "多参数测量数据读取.vi"("探头选择"=w342) -> ("error out"=w331:errorcluster, "测量数据块"=w336:T5)  [unwired: 8 in, 1 out]
                  n180 = case shown="无错误" w331 {
                    tunnel: w336 -> [w343 _]
                    frame No Error {
                      n181 = global write "多参数全局变量.vi" "叶绿素数据区"(w343) -> ()
                    }
                    frame Error {
                    }
                  }
                  n182 = call "多参数据转列表.vi"("参数名"="叶绿素a", "测量数据块"=w336) -> ("添加的数组"=w334:string[][])  [unwired: 9 in]
                  n183 = Index Array(array=w334) -> (element #1=w333:string[], element #2=w332:string[])  [unwired: 4 in]
                  n184 = Insert Into Array(array=w341, new element=w332) -> (w340:string[][])  [unwired: 2 in]
                }
                frame 15 {
                  w355 = u16 15 items=["氨氮"=3, "水温"=9, "pH"=10, "溶解氧"=11, "电导率"=12, "浊度"=13, "叶绿素a"=14, "藻密度"=15, "蓝绿藻"=16, "氧化还原电位"=17, "溶解氧%"=18, "盐度"=19, "水中油"=20, "高锰酸盐指数"=21, "化学需氧量"=22, "比电导率"=23, "总溶解固体"=24, "pH电极电位"=25] ("下拉列表")
                  n185 = call "多参数测量数据读取.vi"("探头选择"=w355) -> ("error out"=w344:errorcluster, "测量数据块"=w347:T5)  [unwired: 8 in, 1 out]
                  n186 = case shown="无错误" w344 {
                    tunnel: w347 -> [w356 _]
                    frame No Error {
                      n187 = global write "多参数全局变量.vi" "藻密度数据区"(w356) -> ()
                    }
                    frame Error {
                    }
                  }
                  n188 = call "多参数据转列表.vi"("参数名"="藻密度", "测量数据块"=w347) -> ("添加的数组"=w349:string[][])  [unwired: 9 in]
                  n189 = Index Array(array=w349) -> (element #1=w348:string[], element #2=w346:string[])  [unwired: 4 in]
                  n190 = Insert Into Array(array=w354, new element=w346) -> (w353:string[][])  [unwired: 2 in]
                  n191 = Bundle By Name(cluster=w351, "藻密度"=1.0 ("DO")) -> (w350:T10)
                }
                frame 16 {
                  w368 = u16 16 items=["氨氮"=3, "水温"=9, "pH"=10, "溶解氧"=11, "电导率"=12, "浊度"=13, "叶绿素a"=14, "藻密度"=15, "蓝绿藻"=16, "氧化还原电位"=17, "溶解氧%"=18, "盐度"=19, "水中油"=20, "高锰酸盐指数"=21, "化学需氧量"=22, "比电导率"=23, "总溶解固体"=24, "pH电极电位"=25] ("下拉列表")
                  n192 = call "多参数测量数据读取.vi"("探头选择"=w368) -> ("error out"=w357:errorcluster, "测量数据块"=w362:T5)  [unwired: 8 in, 1 out]
                  n193 = case shown="无错误" w357 {
                    tunnel: w362 -> [w369 _]
                    frame No Error {
                      n194 = global write "多参数全局变量.vi" "蓝绿藻数据区"(w369) -> ()
                    }
                    frame Error {
                    }
                  }
                  n195 = call "多参数据转列表.vi"("参数名"="蓝绿藻", "测量数据块"=w362) -> ("添加的数组"=w361:string[][])  [unwired: 9 in]
                  n196 = Index Array(array=w361) -> (element #1=w360:string[], element #2=w359:string[])  [unwired: 4 in]
                  n197 = Insert Into Array(array=w367, new element=w359) -> (w366:string[][])  [unwired: 2 in]
                  n198 = Bundle By Name(cluster=w364, "蓝绿藻"=1.0 ("DO")) -> (w363:T10)
                }
                frame 17 {
                  w381 = u16 17 items=["氨氮"=3, "水温"=9, "pH"=10, "溶解氧"=11, "电导率"=12, "浊度"=13, "叶绿素a"=14, "藻密度"=15, "蓝绿藻"=16, "氧化还原电位"=17, "溶解氧%"=18, "盐度"=19, "水中油"=20, "高锰酸盐指数"=21, "化学需氧量"=22, "比电导率"=23, "总溶解固体"=24, "pH电极电位"=25] ("下拉列表")
                  n199 = Bundle By Name(cluster=w377, "ORP"=1.0 ("DO")) -> (w376:T10)
                  n200 = call "多参数测量数据读取.vi"("探头选择"=w381) -> ("error out"=w370:errorcluster, "测量数据块"=w375:T5)  [unwired: 8 in, 1 out]
                  n201 = case shown="无错误" w370 {
                    tunnel: w375 -> [w382 _]
                    frame No Error {
                      n202 = global write "多参数全局变量.vi" "ORP数据区"(w382) -> ()
                    }
                    frame Error {
                    }
                  }
                  n203 = call "多参数据转列表.vi"("参数名"="ORP", "测量数据块"=w375) -> ("添加的数组"=w374:string[][])  [unwired: 9 in]
                  n204 = Index Array(array=w374) -> (element #1=w373:string[], element #2=w371:string[])  [unwired: 4 in]
                  n205 = Insert Into Array(array=w380, new element=w371) -> (w379:string[][])  [unwired: 2 in]
                }
                frame 20 {
                  w391 = u16 20 items=["氨氮"=3, "水温"=9, "pH"=10, "溶解氧"=11, "电导率"=12, "浊度"=13, "叶绿素a"=14, "藻密度"=15, "蓝绿藻"=16, "氧化还原电位"=17, "溶解氧%"=18, "盐度"=19, "水中油"=20, "高锰酸盐指数"=21, "化学需氧量"=22, "比电导率"=23, "总溶解固体"=24, "pH电极电位"=25] ("下拉列表")
                  n206 = call "多参数测量数据读取.vi"("探头选择"=w391) -> ("测量数据块"=w387:T5)  [unwired: 8 in, 2 out]
                  n207 = call "多参数据转列表.vi"("参数名"="水中油", "测量数据块"=w387) -> ("添加的数组"=w385:string[][])  [unwired: 9 in]
                  n208 = Index Array(array=w385) -> (element #1=w384:string[], element #2=w383:string[])  [unwired: 4 in]
                  n209 = Insert Into Array(array=w390, new element=w383) -> (w389:string[][])  [unwired: 2 in]
                }
                frame 21 {
                  w400 = u16 21 items=["氨氮"=3, "水温"=9, "pH"=10, "溶解氧"=11, "电导率"=12, "浊度"=13, "叶绿素a"=14, "藻密度"=15, "蓝绿藻"=16, "氧化还原电位"=17, "溶解氧%"=18, "盐度"=19, "水中油"=20, "高锰酸盐指数"=21, "化学需氧量"=22, "比电导率"=23, "总溶解固体"=24, "pH电极电位"=25] ("下拉列表")
                  n210 = call "多参数测量数据读取.vi"("探头选择"=w400) -> ("测量数据块"=w396:T5)  [unwired: 8 in, 2 out]
                  n211 = call "多参数据转列表.vi"("参数名"="高锰酸盐指数", "测量数据块"=w396) -> ("添加的数组"=w395:string[][])  [unwired: 9 in]
                  n212 = Index Array(array=w395) -> (element #1=w393:string[], element #2=w392:string[])  [unwired: 4 in]
                  n213 = Insert Into Array(array=w399, new element=w392) -> (w398:string[][])  [unwired: 2 in]
                }
                frame 22 {
                  w409 = u16 22 items=["氨氮"=3, "水温"=9, "pH"=10, "溶解氧"=11, "电导率"=12, "浊度"=13, "叶绿素a"=14, "藻密度"=15, "蓝绿藻"=16, "氧化还原电位"=17, "溶解氧%"=18, "盐度"=19, "水中油"=20, "高锰酸盐指数"=21, "化学需氧量"=22, "比电导率"=23, "总溶解固体"=24, "pH电极电位"=25] ("下拉列表")
                  n214 = call "多参数测量数据读取.vi"("探头选择"=w409) -> ("测量数据块"=w405:T5)  [unwired: 8 in, 2 out]
                  n215 = call "多参数据转列表.vi"("参数名"="化学需氧量", "测量数据块"=w405) -> ("添加的数组"=w404:string[][])  [unwired: 9 in]
                  n216 = Index Array(array=w404) -> (element #1=w402:string[], element #2=w401:string[])  [unwired: 4 in]
                  n217 = Insert Into Array(array=w408, new element=w401) -> (w407:string[][])  [unwired: 2 in]
                }
              }
            }
            n218 = global write "多参数全局变量.vi" "传感器通道号"(w183) -> ()
            n219 = property on="数据区" class="MCListbox (严格)"("ColHdrString"=w189, "ItemNames"=w188) -> ()  [unwired: 2 in, 2 out]
          }
          frame Error {
          }
        }
      }
    }
    n220 = Wait (ms)(milliseconds to wait=u32 1000 ("等待时间（毫秒）")) -> ()  [unwired: 1 out]
  }
  n221 = property on="窗格" class="Pane"("Origin"=T3 {"Horizontal"=0, "Vertical"=0} ("原点")) -> ()  [unwired: 2 in, 2 out]
  n222 = property class="VI"(reference=w8) -> ("Library.Version"=w7:T11)  [unwired: 1 in, 2 out]
  n223 = call <vilib>:"Application Directory.vi"() -> ("Application Directory"=w14:path)
  n224 = Build Path(base path=w14, name or relative path="data\\sys.ini" ("名称或相对路径")) -> (appended path=w16:path)
  n225 = Unbundle By Name(w7) -> ("Major"=w5:u16, "Minor"=w4:u16, "Fix"=w3:u16, "Build"=w2:u16)
  n226 = call <vilib>:"Open Config Data.vi"("configuration file path"=w16) -> ("error out"=w20:errorcluster, "refnum"=w17:T12)  [unwired: 8 in, 1 out]
  n227 = vi-ref "多参数断电保存全局变量.vi"() -> (w18:refnum<vi>)
  n228 = call <userlib>:"Read Panel from INI__ogtk.vi"("error in (no error)"=w20, "VI ref"=w18, "refnum"=w17) -> ("error out"=w21:errorcluster, "refnum out"=w19:T12)  [unwired: 7 in]
  n229 = Obtain Queue(name (unnamed)="Mp Task" ("名称（未命名）"), element data type=T2 {"测量模式"=enum."水样测试", "数据类型"="N", "手动启动标记"=FALSE} ("启动参数")) -> (queue out=w9:refnum<queue>)  [unwired: 3 in, 2 out]
  n230 = property on="打开串口" class="Bool (严格)"("Val(Sgnl)"=TRUE ("值(信号)")) -> (error out=w22:errorcluster)  [unwired: 2 in, 1 out]
  n231 = call <vilib>:"Close Config Data.vi"("error in (no error)"=w21, "refnum"=w19) -> ("error out"=w13:errorcluster)  [unwired: 8 in, 1 out]
  n232 = Format Into String(format string="模块版本号：%d.%d.%d.%d" ("格式字符串"), w5, w4, w3, w2) -> (resulting string=→"模块版本号":string)  [unwired: 2 in, 1 out]
  n233 = Obtain Notifier(name (unnamed)="MPFlow" ("名称（未命名）"), notification data type=FALSE) -> (notifier out=w25:refnum<notifier>)  [unwired: 2 in, 2 out]
  n234 = while {
    tunnel: w9 -> [w411]
    stop <- FALSE stop-if-true
    n235 = flat-sequence {
      tunnel: w411 -> [w415]
      tunnel: [w413] -> w410
      frame #0 {
        n236 = Dequeue Element(queue=w415) -> (queue out=w413:refnum<queue>, element=w414:T2)  [unwired: 2 in, 2 out]
        n237 = call "五参数水样测试.vi"("启动参数"=w414) -> ()  [unwired: 11 in]
      }
    }
    n238 = Flush Queue(queue=w410) -> ()  [unwired: 1 in, 3 out]
  }
  n239 = vi-ref "斯坦道多参数.lvlib:五参数标样核查.vi"() -> (w12:refnum<vi>)
  n240 = control-ref of="控制命令区探头选择"() -> (w24:refnum<vi>)
  n241 = while {
    tunnel: w25 -> [w419]
    tunnel: w24 -> [w418]
    tunnel: w22 -> [_]
    tunnel: w13 -> [_]
    tunnel: w12 -> [w417]
    tunnel: w9 -> [w416]
    stop <- FALSE stop-if-true
    n242 = event shown="[6] \"串口设置\": 值改变" {
      selector: _ -> [_ _ _ _ _ _ _ _ _ _ _ _ _ _ _ _ _ _ _ _ _ _ _ _ _ _]
      dyn-events: _ -> [_ _ _ _ _ _ _ _ _ _ _ _ _ _ _ _ _ _ _ _ _ _ _ _ _ _]
      timeout: _ -> [_ _ _ _ _ _ _ _ _ _ _ _ _ _ _ _ _ _ _ _ _ _ _ _ _ _]
      tunnel: w419 -> [_ _ _ _ _ _ _ _ _ _ _ _ _ _ _ w607 _ _ _ _ _ _ _ _ _ _]
      tunnel: w418 -> [_ _ w428 w432 _ _ _ _ _ _ _ _ _ _ _ _ _ _ _ _ _ _ _ _ w664 w671]
      tunnel: w417 -> [_ _ _ _ _ _ _ _ _ _ _ _ _ _ w583 _ _ _ _ _ _ _ _ _ _ _]
      tunnel: w416 -> [_ _ _ _ _ _ _ _ _ _ _ _ _ w579 _ _ _ _ _ _ _ _ _ _ _ _]
      event Timeout {
        n243 = event-data() -> ()  [unwired: 1 in, 3 out]
      }
      event "K", "B", "水深校准", "水样稳定时间", "上电初始化时间", "转刷清洗时间", "水样测试组数", "标样测试组数": Mouse Down {
        n244 = event-data() -> ("CtlRef"=w424:refnum<vi>)  [unwired: 1 in, 7 out]
        n245 = property class="DigNum (严格)"(reference=w424) -> (reference out=w422:refnum<vi>, "Value"=w423:dbl)  [unwired: 1 in, 1 out]
        n246 = call "数字键盘.vi"("OldNumber"=w423) -> ("NewNumber"=w421:dbl)
        n247 = property class="DigNum (严格)"(reference=w422, "Value"=w421) -> ()  [unwired: 1 in, 2 out]
      }
      event "读取": Value Change {
        n248 = event-data() -> ()  [unwired: 1 in, 6 out]
        n249 = property class="Ring (严格)"(reference=w428) -> ("Value"=w427:u16)  [unwired: 1 in, 2 out]
        n250 = call "多参校准读取.vi"("站号"=w427) -> ("B"=w425:dbl, "K"=w426:dbl)  [unwired: 8 in, 1 out]
        n251 = local write "K"(w426) -> ()
        n252 = local write "B"(w425) -> ()
      }
      event "写入": Value Change {
        n253 = event-data() -> ()  [unwired: 1 in, 6 out]
        n254 = property class="Ring (严格)"(reference=w432) -> ("Value"=w431:u16)  [unwired: 1 in, 2 out]
        n255 = call "多参数校准写入.vi"("B"="B", "K"="K", "站号"=w431) -> ()  [unwired: 8 in, 1 out]
      }
      event "水深读取": Value Change {
        w434 = u16 9 items=["氨氮"=3, "水温"=9, "pH值"=10, "溶解氧"=11, "电导率"=12, "浊度"=13, "叶绿素a"=14, "藻密度"=15, "蓝绿藻"=16, "氧化还原电位"=17, "溶解氧%"=18, "盐度"=19] ("站号")
        n256 = event-data() -> ()  [unwired: 1 in, 6 out]
        n257 = call "多参水深校准读取.vi"("站号"=w434) -> ("B"=w433:dbl)  [unwired: 8 in, 2 out]
        n258 = local write "水深校准"(w433) -> ()
      }
      event "水深写入": Value Change {
        w436 = u16 9 items=["氨氮"=3, "水温"=9, "pH值"=10, "溶解氧"=11, "电导率"=12, "浊度"=13, "叶绿素a"=14, "藻密度"=15, "蓝绿藻"=16, "氧化还原电位"=17, "溶解氧%"=18, "盐度"=19] ("站号")
        n259 = event-data() -> ()  [unwired: 1 in, 6 out]
        n260 = call "多参数水深校准写入.vi"("K"="水深校准", "站号"=w436) -> ()  [unwired: 9 in, 1 out]
      }
      event "串口设置": Value Change {
        n261 = event-data() -> ()  [unwired: 1 in, 6 out]
        n262 = global read "多参数断电保存全局变量.vi" "VISA Resource"() -> (w441:refnum<visa-resource-name>)
        n263 = global read "多参数断电保存全局变量.vi" "波特率"() -> (w439:u32)
        n264 = call "串口配置.vi"("波特率"=w439, "VISA资源名称"=w441) -> ("确认 2"=w437:bool, "波特率 2"=w438:u32, "VISA资源名称 2"=w440:refnum<visa-resource-name>)  [unwired: 7 in]
        n265 = case shown="真" w437 {
          tunnel: w440 -> [_ w443]
          tunnel: w438 -> [_ w442]
          frame False {
          }
          frame True {
            n266 = flat-sequence {
              tunnel: w443 -> [w445]
              tunnel: w442 -> [w444]
              frame #0 {
                n267 = global write "多参数断电保存全局变量.vi" "波特率"(w444) -> ()
                n268 = global write "多参数断电保存全局变量.vi" "VISA Resource"(w445) -> ()
              }
              frame #1 {
                n269 = call "多参数通讯.vi"("STEP"=enum16{"open", "read", "write", "close"}."open") -> ("error out"=w447:errorcluster)  [unwired: 8 in, 2 out]
                n270 = case shown="错误" w447 {
                  frame No Error {
                  }
                  frame Error {
                    n271 = One Button Dialog(message="多参数串口打开失败" ("消息")) -> ()  [unwired: 1 in, 1 out]
                  }
                }
              }
              frame #2 {
                n272 = call <vilib>:"Application Directory.vi"() -> ("Application Directory"=w462:path)
                n273 = Build Path(base path=w462, name or relative path="data\\sys.ini" ("名称或相对路径")) -> (appended path=w460:path)
                n274 = call <vilib>:"Open Config Data.vi"("configuration file path"=w460) -> ("error out"=w456:errorcluster, "refnum"=w459:T12)  [unwired: 8 in, 1 out]
                n275 = vi-ref "多参数断电保存全局变量.vi"() -> (w458:refnum<vi>)
                n276 = call <userlib>:"Write Panel to INI__ogtk.vi"("error in (no error)"=w456, "VI ref"=w458, "refnum"=w459) -> ("error out"=w455:errorcluster, "refnum out"=w457:T12)  [unwired: 7 in]
                n277 = call <vilib>:"Close Config Data.vi"("error in (no error)"=w455, "refnum"=w457) -> ("error out"=w450:errorcluster, "file path"=w449:path)  [unwired: 8 in]
                n278 = Open/Create/Replace File(file path (use dialog)=w449, error in=w450) -> (refnum out=w453:refnum<file>, error out=w454:errorcluster)  [unwired: 4 in, 1 out]
                n279 = Flush File(refnum=w453, error in=w454) -> (refnum out=w452:refnum<file>, error out=w451:errorcluster)
                n280 = Close File(refnum=w452, error in=w451) -> ()  [unwired: 2 out]
              }
            }
          }
        }
      }
      event "水样稳定时间", "上电初始化时间", "转刷清洗时间", "水样测试组数", "标样测试组数": Value Change {
        n281 = event-data() -> ()  [unwired: 1 in, 6 out]
        n282 = flat-sequence {
          frame #0 {
            n283 = global write "多参数断电保存全局变量.vi" "水样稳定时间"("水样稳定时间") -> ()
            n284 = global write "多参数断电保存全局变量.vi" "水样测试组数"("水样测试组数") -> ()
            n285 = global write "多参数断电保存全局变量.vi" "上电初始化时间"("上电初始化时间") -> ()
            n286 = global write "多参数断电保存全局变量.vi" "转刷清洗时间"("转刷清洗时间") -> ()
            n287 = global write "多参数断电保存全局变量.vi" "标样测试组数"("标样测试组数") -> ()
          }
          frame #1 {
            n288 = call <vilib>:"Application Directory.vi"() -> ("Application Directory"=w481:path)
            n289 = Build Path(base path=w481, name or relative path="data\\sys.ini" ("名称或相对路径")) -> (appended path=w479:path)
            n290 = call <vilib>:"Open Config Data.vi"("configuration file path"=w479) -> ("error out"=w475:errorcluster, "refnum"=w478:T12)  [unwired: 8 in, 1 out]
            n291 = vi-ref "多参数断电保存全局变量.vi"() -> (w477:refnum<vi>)
            n292 = call <userlib>:"Write Panel to INI__ogtk.vi"("error in (no error)"=w475, "VI ref"=w477, "refnum"=w478) -> ("error out"=w474:errorcluster, "refnum out"=w476:T12)  [unwired: 7 in]
            n293 = call <vilib>:"Close Config Data.vi"("error in (no error)"=w474, "refnum"=w476) -> ("error out"=w469:errorcluster, "file path"=w468:path)  [unwired: 8 in]
            n294 = Open/Create/Replace File(file path (use dialog)=w468, error in=w469) -> (refnum out=w472:refnum<file>, error out=w473:errorcluster)  [unwired: 4 in, 1 out]
            n295 = Flush File(refnum=w472, error in=w473) -> (refnum out=w471:refnum<file>, error out=w470:errorcluster)
            n296 = Close File(refnum=w471, error in=w470) -> ()  [unwired: 2 out]
          }
        }
      }
      event "传感器参数自动获取": Value Change {
        n297 = event-data() -> ("NewVal"=w482:bool)  [unwired: 1 in, 5 out]
        n298 = case shown="假" w482 {
          frame False {
            n299 = property on="获取传感器参数并保存触发" class="Bool (严格)"("Val(Sgnl)"=FALSE ("获取传感器参数并保存触发")) -> ()  [unwired: 2 in, 2 out]
          }
          frame True {
          }
        }
        n300 = flat-sequence {
          tunnel: w482 -> [w484]
          frame #0 {
            n301 = global write "多参数断电保存全局变量.vi" "传感器参数自动获取"(w484) -> ()
          }
          frame #1 {
            n302 = call <vilib>:"Application Directory.vi"() -> ("Application Directory"=w498:path)
            n303 = Build Path(base path=w498, name or relative path="data\\sys.ini" ("名称或相对路径")) -> (appended path=w496:path)
            n304 = call <vilib>:"Open Config Data.vi"("configuration file path"=w496) -> ("error out"=w492:errorcluster, "refnum"=w495:T12)  [unwired: 8 in, 1 out]
            n305 = vi-ref "多参数断电保存全局变量.vi"() -> (w494:refnum<vi>)
            n306 = call <userlib>:"Write Panel to INI__ogtk.vi"("error in (no error)"=w492, "VI ref"=w494, "refnum"=w495) -> ("error out"=w491:errorcluster, "refnum out"=w493:T12)  [unwired: 7 in]
            n307 = call <vilib>:"Close Config Data.vi"("error in (no error)"=w491, "refnum"=w493) -> ("error out"=w486:errorcluster, "file path"=w485:path)  [unwired: 8 in]
            n308 = Open/Create/Replace File(file path (use dialog)=w485, error in=w486) -> (refnum out=w489:refnum<file>, error out=w490:errorcluster)  [unwired: 4 in, 1 out]
            n309 = Flush File(refnum=w489, error in=w490) -> (refnum out=w488:refnum<file>, error out=w487:errorcluster)
            n310 = Close File(refnum=w488, error in=w487) -> ()  [unwired: 2 out]
          }
        }
      }
      event "质控参数设置": Value Change {
        n311 = event-data() -> ()  [unwired: 1 in, 6 out]
        n312 = global read "多参数断电保存全局变量.vi" "质控参数设置"() -> (w499:T15)
        n313 = call "多参数质控参数设置.vi"("质控参数设置"=w499) -> ("输出簇"=w500:T16)  [unwired: 10 in]
        n314 = Unbundle By Name(w500) -> ("确定"=w501:bool)
        n315 = case shown="真" w501 {
          tunnel: w500 -> [_ w503]
          tunnel: w499 -> [_ w502]
          frame False {
          }
          frame True {
            n316 = flat-sequence {
              tunnel: w503 -> [w511]
              tunnel: w502 -> [w510]
              frame #0 {
                n317 = Unbundle By Name(w511) -> ("水温标准液标准浓度"=w509:dbl, "酸碱度标准液标准浓度"=w508:dbl, "溶解氧标准液标准浓度"=w507:dbl, "电导率标准液标准浓度"=w506:dbl, "浊度标准液标准浓度"=w505:dbl)
                n318 = Bundle By Name(cluster=w510, "水温标准液标准浓度"=w509, "酸碱度标准液标准浓度"=w508, "溶解氧标准液标准浓度"=w507, "电导率标准液标准浓度"=w506, "浊度标准液标准浓度"=w505) -> (w504:T15)
                n319 = global write "多参数断电保存全局变量.vi" "质控参数设置"(w504) -> ()
              }
              frame #1 {
                n320 = call <vilib>:"Application Directory.vi"() -> ("Application Directory"=w525:path)
                n321 = Build Path(base path=w525, name or relative path="data\\sys.ini" ("名称或相对路径")) -> (appended path=w523:path)
                n322 = call <vilib>:"Open Config Data.vi"("configuration file path"=w523) -> ("error out"=w519:errorcluster, "refnum"=w522:T12)  [unwired: 8 in, 1 out]
                n323 = vi-ref "多参数断电保存全局变量.vi"() -> (w521:refnum<vi>)
                n324 = call <userlib>:"Write Panel to INI__ogtk.vi"("error in (no error)"=w519, "VI ref"=w521, "refnum"=w522) -> ("error out"=w518:errorcluster, "refnum out"=w520:T12)  [unwired: 7 in]
                n325 = call <vilib>:"Close Config Data.vi"("error in (no error)"=w518, "refnum"=w520) -> ("error out"=w513:errorcluster, "file path"=w512:path)  [unwired: 8 in]
                n326 = Open/Create/Replace File(file path (use dialog)=w512, error in=w513) -> (refnum out=w516:refnum<file>, error out=w517:errorcluster)  [unwired: 4 in, 1 out]
                n327 = Flush File(refnum=w516, error in=w517) -> (refnum out=w515:refnum<file>, error out=w514:errorcluster)
                n328 = Close File(refnum=w515, error in=w514) -> ()  [unwired: 2 out]
              }
            }
          }
        }
      }
      event "仪器参数设置": Value Change {
        n329 = event-data() -> ()  [unwired: 1 in, 6 out]
        n330 = global read "多参数断电保存全局变量.vi" "PH参数"() -> (w535:T4)
        n331 = global read "多参数断电保存全局变量.vi" "电导率参数"() -> (w534:T4)
        n332 = global read "多参数断电保存全局变量.vi" "溶解氧参数"() -> (w533:T4)
        n333 = global read "多参数断电保存全局变量.vi" "水温参数"() -> (w532:T4)
        n334 = global read "多参数断电保存全局变量.vi" "浊度参数"() -> (w531:T4)
        n335 = global read "多参数断电保存全局变量.vi" "叶绿素参数"() -> (w530:T4)
        n336 = global read "多参数断电保存全局变量.vi" "藻密度参数"() -> (w528:T4)
        n337 = global read "多参数断电保存全局变量.vi" "ORP参数"() -> (w529:T4)
        n338 = Build Array(w535, w534, w533, w532, w531, w530, w528, w529) -> (w527:T6)
        n339 = call "仪器参数设置.vi"("仪器参数设置输入"=w527) -> ("确定"=w536:bool, "仪器参数设置输出"=w526:T6)  [unwired: 9 in]
        n340 = case shown="真" w536 {
          tunnel: w526 -> [_ w537]
          frame False {
          }
          frame True {
            n341 = flat-sequence {
              tunnel: w537 -> [w546]
              frame #0 {
                n342 = Index Array(array=w546) -> (element #1=w545:T4, element #2=w544:T4, element #3=w543:T4, element #4=w542:T4, element #5=w541:T4, element #6=w538:T4, element #7=w539:T4, element #8=w540:T4)  [unwired: 8 in]
                n343 = global write "多参数断电保存全局变量.vi" "PH参数"(w545) -> ()
                n344 = global write "多参数断电保存全局变量.vi" "电导率参数"(w544) -> ()
                n345 = global write "多参数断电保存全局变量.vi" "溶解氧参数"(w543) -> ()
                n346 = global write "多参数断电保存全局变量.vi" "水温参数"(w542) -> ()
                n347 = global write "多参数断电保存全局变量.vi" "浊度参数"(w541) -> ()
                n348 = global write "多参数断电保存全局变量.vi" "叶绿素参数"(w538) -> ()
                n349 = global write "多参数断电保存全局变量.vi" "藻密度参数"(w539) -> ()
                n350 = global write "多参数断电保存全局变量.vi" "ORP参数"(w540) -> ()
              }
              frame #1 {
                n351 = call <vilib>:"Application Directory.vi"() -> ("Application Directory"=w560:path)
                n352 = Build Path(base path=w560, name or relative path="data\\sys.ini" ("名称或相对路径")) -> (appended path=w558:path)
                n353 = call <vilib>:"Open Config Data.vi"("configuration file path"=w558) -> ("error out"=w554:errorcluster, "refnum"=w557:T12)  [unwired: 8 in, 1 out]
                n354 = vi-ref "多参数断电保存全局变量.vi"() -> (w556:refnum<vi>)
                n355 = call <userlib>:"Write Panel to INI__ogtk.vi"("error in (no error)"=w554, "VI ref"=w556, "refnum"=w557) -> ("error out"=w553:errorcluster, "refnum out"=w555:T12)  [unwired: 7 in]
                n356 = call <vilib>:"Close Config Data.vi"("error in (no error)"=w553, "refnum"=w555) -> ("error out"=w548:errorcluster, "file path"=w547:path)  [unwired: 8 in]
                n357 = Open/Create/Replace File(file path (use dialog)=w547, error in=w548) -> (refnum out=w551:refnum<file>, error out=w552:errorcluster)  [unwired: 4 in, 1 out]
                n358 = Flush File(refnum=w551, error in=w552) -> (refnum out=w550:refnum<file>, error out=w549:errorcluster)
                n359 = Close File(refnum=w550, error in=w549) -> ()  [unwired: 2 out]
              }
            }
          }
        }
      }
      event "释放串口": Value Change {
        n360 = event-data() -> ("NewVal"=w561:bool)  [unwired: 1 in, 5 out]
        n361 = case shown="真" w561 {
          frame False {
          }
          frame True {
            n362 = call "多参数通讯.vi"("STEP"=enum16{"open", "read", "write", "close"}."close") -> ("error out"=w562:errorcluster)  [unwired: 8 in, 2 out]
            n363 = case shown="无错误" w562 {
              frame No Error {
                n364 = property on="打开串口" class="Bool (严格)"("DisabledEnum"=T13."Enabled" ("禁用")) -> ()  [unwired: 2 in, 2 out]
              }
              frame Error {
              }
            }
          }
        }
      }
      event "打开串口": Value Change {
        n365 = event-data() -> ("NewVal"=w565:bool)  [unwired: 1 in, 5 out]
        n366 = case shown="真" w565 {
          frame False {
          }
          frame True {
            n367 = call "多参数通讯.vi"("STEP"=enum16{"open", "read", "write", "close"}."open") -> ("error out"=w566:errorcluster)  [unwired: 8 in, 2 out]
            n368 = case shown="错误" w566 {
              tunnel: [T13."Disabled and Grayed Out" ("禁用") T13."Enabled" ("禁用")] -> w568
              frame No Error {
              }
              frame Error {
                n369 = One Button Dialog(message="多参数串口打开失败" ("消息")) -> ()  [unwired: 1 in, 1 out]
              }
            }
            n370 = property on="打开串口" class="Bool (严格)"("DisabledEnum"=w568, "Value"=FALSE ("打开串口")) -> ()  [unwired: 2 in, 2 out]
          }
        }
      }
      event "水样测试": Value Change {
        n371 = event-data() -> ()  [unwired: 1 in, 6 out]
        n372 = global read "多参数断电保存全局变量.vi" "运行周期"() -> (w575:T17)
        n373 = Unbundle By Name(w575) -> ("运行模式"=w574:enum16{"维护模式", "常规模式", "应急模式", "质控模式"})
        n374 = case shown="\"常规模式\", 默认" w574 {
          tunnel: ["M" ("数据标记表") "N" ("数据标记表")] -> w578
          frame "维护模式" {
          }
          frame "常规模式", Default {
          }
        }
        n375 = Bundle By Name(cluster=T2 {"测量模式"=enum."水样测试", "数据类型"="N", "手动启动标记"=FALSE} ("启动参数"), "数据类型"=w578, "手动启动标记"=TRUE) -> (w573:T2)
        n376 = Enqueue Element(queue=w579, element=w573) -> ()  [unwired: 2 in, 3 out]
      }
      event "标样核查": Value Change {
        n377 = event-data() -> ()  [unwired: 1 in, 6 out]
        n378 = call "多参数标样核查对话框.vi"() -> ("确认"=w584:bool, "输出参数"=w582:T18)  [unwired: 10 in]
        n379 = case shown="真" w584 {
          tunnel: w583 -> [_ w587]
          tunnel: w582 -> [_ w586]
          frame False {
          }
          frame True {
            n380 = property class="VI"(reference=w587) -> ("Name"=w591:string, "Exec.State"=w589:T19)  [unwired: 1 in, 2 out]
            n381 = Open VI Reference(type specifier VI Refnum (for type only)=refnum<vi> refnum, vi path=w591, options=128 ("选项")) -> (vi reference=w590:refnum<vi>)  [unwired: 3 in, 1 out]
            n382 = case shown="\"Idle\"" w589 {
              tunnel: w590 -> [w594 w602]
              tunnel: [w594 w601] -> w588
              tunnel: w586 -> [_ w598]
              frame "Bad", Default {
                n383 = One Button Dialog(message="仪器已经启动，无需重复启动" ("消息")) -> ()  [unwired: 1 in, 1 out]
              }
              frame "Idle" {
                n384 = global read "多参数断电保存全局变量.vi" "运行周期"() -> (w596:T17)
                n385 = Unbundle By Name(w596) -> ("运行模式"=w595:enum16{"维护模式", "常规模式", "应急模式", "质控模式"})
                n386 = case shown="\"常规模式\", 默认" w595 {
                  tunnel: ["M" ("数据标记表") "N" ("数据标记表")] -> w600
                  frame "维护模式" {
                  }
                  frame "常规模式", Default {
                  }
                }
                n387 = Bundle By Name(cluster=T14 {"测量模式"=enum."标样核查", "数据标记表"="N", "输出参数"={"水温"=FALSE, "pH"=FALSE, "DO"=FALSE, "浊度"=FALSE, "电导率"=FALSE}} ("启动参数"), "数据标记表"=w600, "输出参数"=w598) -> (w599:T14)
                n388 = call-by-ref "开始异步调用"(reference=w602, "启动参数"=w599) -> (reference out=w601:refnum<vi>)  [unwired: 12 in, 1 out]
              }
            }
            n389 = Close Reference(reference=w588) -> ()  [unwired: 1 in, 1 out]
          }
        }
      }
      event "停止": Value Change {
        n390 = event-data() -> ()  [unwired: 1 in, 6 out]
        n391 = Two Button Dialog(message="请再一次确认是否停止测量" ("消息")) -> (T button?=w605:bool)  [unwired: 2 in]
        n392 = case shown="真" w605 {
          tunnel: w607 -> [_ w610]
          frame False {
          }
          frame True {
            w608 = u16 11 items=["启动测量（全部）"=1, "初始化（清洗）"=10, "停止测量（全部）"=11, "校时"=13, "启动测量（单个传感器）"=19, "停止测量（单个传感器）"=20] ("控制命令")
            w609 = u16 10 items=["氨氮"=3, "水温"=9, "pH值"=10, "溶解氧"=11, "电导率"=12, "浊度"=13, "叶绿素a"=14, "藻密度"=15, "蓝绿藻"=16, "氧化还原电位"=17, "溶解氧%"=18, "盐度"=19] ("站号")
            n393 = Send Notification(notification=TRUE ("通知"), notifier=w610) -> ()  [unwired: 1 in, 2 out]
            n394 = call "多参数控制命令.vi"("控制命令"=w608, "站号"=w609) -> ()  [unwired: 9 in, 1 out]
          }
        }
      }
      event "设置": Value Change {
        n395 = event-data() -> ()  [unwired: 1 in, 6 out]
        n396 = property on="窗格" class="Pane"("Origin"=T3 {"Horizontal"=0, "Vertical"=628} ("原点")) -> ()  [unwired: 2 in, 2 out]
      }
      event "返回": Value Change {
        n397 = event-data() -> ()  [unwired: 1 in, 6 out]
        n398 = property on="窗格" class="Pane"("Origin"=T3 {"Horizontal"=0, "Vertical"=0} ("原点")) -> ()  [unwired: 2 in, 2 out]
      }
      event "传感器参数读取", "获取传感器参数并保存触发": Value Change {
        n399 = event-data() -> ()  [unwired: 1 in, 6 out]
        n400 = call "多参数传感器参数读取.vi"() -> ("error out"=w617:errorcluster, "modbus"=w615:u16[], "添加的数组"=w616:string[][])  [unwired: 9 in]
        n401 = property on="传感器区" class="MCListbox (严格)"("ItemNames"=w616) -> ()  [unwired: 2 in, 2 out]
        n402 = call <vilib>:"General Error Handler.vi"("error in (no error)"=w617) -> ("error out"=w614:errorcluster)  [unwired: 10 in, 4 out]
        n403 = case shown="无错误" w614 {
          tunnel: w615 -> [w618 _]
          frame No Error {
            n404 = flat-sequence {
              tunnel: w618 -> [w619]
              frame #0 {
                n405 = global write "多参数断电保存全局变量.vi" "传感器参数modbus"(w619) -> ()
              }
              frame #1 {
                n406 = call <vilib>:"Application Directory.vi"() -> ("Application Directory"=w633:path)
                n407 = Build Path(base path=w633, name or relative path="data\\sys.ini" ("名称或相对路径")) -> (appended path=w631:path)
                n408 = call <vilib>:"Open Config Data.vi"("configuration file path"=w631) -> ("error out"=w627:errorcluster, "refnum"=w630:T12)  [unwired: 8 in, 1 out]
                n409 = vi-ref "多参数断电保存全局变量.vi"() -> (w629:refnum<vi>)
                n410 = call <userlib>:"Write Panel to INI__ogtk.vi"("error in (no error)"=w627, "VI ref"=w629, "refnum"=w630) -> ("error out"=w626:errorcluster, "refnum out"=w628:T12)  [unwired: 7 in]
                n411 = call <vilib>:"Close Config Data.vi"("error in (no error)"=w626, "refnum"=w628) -> ("error out"=w621:errorcluster, "file path"=w620:path)  [unwired: 8 in]
                n412 = Open/Create/Replace File(file path (use dialog)=w620, error in=w621) -> (refnum out=w624:refnum<file>, error out=w625:errorcluster)  [unwired: 4 in, 1 out]
                n413 = Flush File(refnum=w624, error in=w625) -> (refnum out=w623:refnum<file>, error out=w622:errorcluster)
                n414 = Close File(refnum=w623, error in=w622) -> ()  [unwired: 2 out]
              }
            }
          }
          frame Error {
          }
        }
      }
      event "关键参数区读取": Value Change {
        n415 = event-data() -> ()  [unwired: 1 in, 6 out]
        n416 = call "多参数关键参数读取.vi"() -> ("error out"=w634:errorcluster, "添加的数组"=w635:string[][])  [unwired: 10 in]
        n417 = property on="关键参数区" class="MCListbox (严格)"("ItemNames"=w635) -> ()  [unwired: 2 in, 2 out]
        n418 = call <vilib>:"General Error Handler.vi"("error in (no error)"=w634) -> ()  [unwired: 10 in, 5 out]
      }
      event "同步时间": Value Change {
        w636 = u16 13 items=["启动测量（全部）"=1, "初始化（清洗）"=10, "停止测量（全部）"=11, "校时"=13, "启动测量（单个传感器）"=19, "停止测量（单个传感器）"=20] ("控制命令")
        w637 = u16 9 items=["氨氮"=3, "水温"=9, "pH值"=10, "溶解氧"=11, "电导率"=12, "浊度"=13, "叶绿素a"=14, "藻密度"=15, "蓝绿藻"=16, "氧化还原电位"=17, "溶解氧%"=18, "盐度"=19] ("站号")
        n419 = event-data() -> ()  [unwired: 1 in, 6 out]
        n420 = call "多参数控制命令.vi"("控制命令"=w636, "站号"=w637) -> ("error out"=w639:errorcluster)  [unwired: 9 in]
        n421 = case shown="错误" w639 {
          tunnel: ["时间同步成功" ("消息") "时间同步失败" ("消息")] -> w638
          frame No Error {
          }
          frame Error {
          }
        }
        n422 = One Button Dialog(message=w638) -> ()  [unwired: 1 in, 1 out]
      }
      event "启动测量(全部)": Value Change {
        w642 = u16 1 items=["启动测量（全部）"=1, "初始化（清洗）"=10, "停止测量（全部）"=11, "校时"=13, "启动测量（单个传感器）"=19, "停止测量（单个传感器）"=20] ("控制命令")
        w643 = u16 9 items=["氨氮"=3, "水温"=9, "pH值"=10, "溶解氧"=11, "电导率"=12, "浊度"=13, "叶绿素a"=14, "藻密度"=15, "蓝绿藻"=16, "氧化还原电位"=17, "溶解氧%"=18, "盐度"=19] ("站号")
        n423 = event-data() -> ()  [unwired: 1 in, 6 out]
        n424 = call "多参数控制命令.vi"("控制命令"=w642, "站号"=w643) -> ("error out"=w645:errorcluster)  [unwired: 9 in]
        n425 = case shown="无错误" w645 {
          tunnel: ["启动成功" ("消息") "启动失败" ("消息")] -> w644
          frame No Error {
          }
          frame Error {
          }
        }
        n426 = One Button Dialog(message=w644) -> ()  [unwired: 1 in, 1 out]
      }
      event "停止测量(全部)": Value Change {
        w650 = u16 11 items=["启动测量（全部）"=1, "初始化（清洗）"=10, "停止测量（全部）"=11, "校时"=13, "启动测量（单个传感器）"=19, "停止测量（单个传感器）"=20] ("控制命令")
        w651 = u16 9 items=["氨氮"=3, "水温"=9, "pH值"=10, "溶解氧"=11, "电导率"=12, "浊度"=13, "叶绿素a"=14, "藻密度"=15, "蓝绿藻"=16, "氧化还原电位"=17, "溶解氧%"=18, "盐度"=19] ("站号")
        n427 = event-data() -> ()  [unwired: 1 in, 6 out]
        n428 = call "多参数控制命令.vi"("控制命令"=w650, "站号"=w651) -> ("error out"=w649:errorcluster)  [unwired: 9 in]
        n429 = case shown="错误" w649 {
          tunnel: ["停止成功" ("消息") "停止失败" ("消息")] -> w648
          frame No Error {
          }
          frame Error {
          }
        }
        n430 = One Button Dialog(message=w648) -> ()  [unwired: 1 in, 1 out]
      }
      event "初始化(清洗)": Value Change {
        w656 = u16 10 items=["启动测量（全部）"=1, "初始化（清洗）"=10, "停止测量（全部）"=11, "校时"=13, "启动测量（单个传感器）"=19, "停止测量（单个传感器）"=20] ("控制命令")
        w657 = u16 9 items=["氨氮"=3, "水温"=9, "pH值"=10, "溶解氧"=11, "电导率"=12, "浊度"=13, "叶绿素a"=14, "藻密度"=15, "蓝绿藻"=16, "氧化还原电位"=17, "溶解氧%"=18, "盐度"=19] ("站号")
        n431 = event-data() -> ()  [unwired: 1 in, 6 out]
        n432 = call "多参数控制命令.vi"("控制命令"=w656, "站号"=w657) -> ("error out"=w654:errorcluster)  [unwired: 9 in]
        n433 = case shown="错误" w654 {
          tunnel: ["初始化成功" ("消息") "初始化失败" ("消息")] -> w655
          frame No Error {
          }
          frame Error {
          }
        }
        n434 = One Button Dialog(message=w655) -> ()  [unwired: 1 in, 1 out]
      }
      event "启动测量(单探)": Value Change {
        w660 = u16 19 items=["启动测量（全部）"=1, "初始化（清洗）"=10, "停止测量（全部）"=11, "校时"=13, "启动测量（单个传感器）"=19, "停止测量（单个传感器）"=20] ("控制命令")
        n435 = event-data() -> ()  [unwired: 1 in, 6 out]
        n436 = property class="Ring (严格)"(reference=w664) -> ("Value"=w663:u16)  [unwired: 1 in, 2 out]
        n437 = call "多参数控制命令.vi"("控制命令"=w660, "站号"=w663) -> ("error out"=w662:errorcluster)  [unwired: 9 in]
        n438 = case shown="无错误" w662 {
          tunnel: ["启动成功" ("消息") "启动失败" ("消息")] -> w661
          frame No Error {
          }
          frame Error {
          }
        }
        n439 = One Button Dialog(message=w661) -> ()  [unwired: 1 in, 1 out]
      }
      event "停止测量(单探)": Value Change {
        w667 = u16 20 items=["启动测量（全部）"=1, "初始化（清洗）"=10, "停止测量（全部）"=11, "校时"=13, "启动测量（单个传感器）"=19, "停止测量（单个传感器）"=20] ("控制命令")
        n440 = event-data() -> ()  [unwired: 1 in, 6 out]
        n441 = property class="Ring (严格)"(reference=w671) -> ("Value"=w670:u16)  [unwired: 1 in, 2 out]
        n442 = call "多参数控制命令.vi"("控制命令"=w667, "站号"=w670) -> ("error out"=w669:errorcluster)  [unwired: 9 in]
        n443 = case shown="错误" w669 {
          tunnel: ["停止成功" ("消息") "停止失败" ("消息")] -> w668
          frame No Error {
          }
          frame Error {
          }
        }
        n444 = One Button Dialog(message=w668) -> ()  [unwired: 1 in, 1 out]
      }
    }
  }
